vi "AU-EGSE Driver.vi"() -> ()   [LabVIEW 2025]
uses:
  <vilib>/Analysis/6fits.llb/Curve Fitting Criteria.ctl
  <vilib>/Analysis/1siggen.llb/Ramp Pattern by Samples.vi
  <vilib>/addons/_JKI Toolkits/State Machine/_JKI_lib_State_Machine.llb/Select State(s)_err__jki_lib_state_machine.vi
  <vilib>/Analysis/1siggen.llb/Ramp Pattern by Delta.vi
  <vilib>/Utility/file.llb/Write Delimited Spreadsheet (string).vi
  <vilib>/Utility/file.llb/Write Delimited Spreadsheet (DBL).vi
  <instrlib>/ULx/ULx_LV.dll
  <vilib>/Analysis/NI_AALBase.lvlib
  <userlib>/_OpenG.lib/time/time.llb/openg_time.lvlib
  <instrlib>/Detector SCPI/Detector SCPI.lvlib
  <instrlib>/Keithley 24XX/Keithley 24XX.lvlib
  <instrlib>/Keithley 648X Series/Keithley 648X Series.lvlib
  <vilib>/Analysis/NI_AALPro.lvlib
panel:
  in  "Exit":bool
  out "Searching":dbl[][](array[numeric])
  in  "Measurement Mode":T1(tab)=enum."SweepCurrent"
  in  "Connect PicoAmmeter":bool
  out "PicoAmmeter Connected":bool
  out "EGSE Connected":bool
  in  "Connect EGSE":bool
  in  "SPI Clock":i64=10000000 format="%^.0e"
  in  "Oversample":i32=1 min=1 max=4096
  in  "Board Power":bool
  in  "Detector VISA":refnum<visa-resource-name>="RS485_Comms"
  out "Voltage (V)":dbl[](array[numeric])=[0.0, 0.0, 0.0, 12.585]
  out "Current (mA)":dbl[](array[numeric])=[0.0, 0.0, 0.0, 0.915]
  in  "ThrowAway":i32=100 min=1 max=10000
  out "Detector EGSE ID String":string
  in  "B2901BL VISA":refnum<visa-resource-name>
  in  "Connect B2901BL":bool
  out "B2901BL Connected":bool
  in  "PicoAmmeter VISA":refnum<visa-resource-name>="Picoammeter"
  out "USB3104 Connected":bool
  in  "USB3104 VOut3 (SWIR)":refnum<k21>="Dev1/Ao3"
  in  "USB3104 VOut5 (MWIR)":refnum<k21>="Dev1/Ao3"
  in  "Connect USB3104":bool
  in  "Heater Power":bool
  in  "Vout3_Res":dbl=9993180.0 format="%#_4p"
  in  "Vout5_Res":dbl=9993180.0 format="%#_5p"
  in  "Set_SWIR":bool
  in  "MWIR Current":dbl
  in  "SWIR Current":dbl
  in  "ContGraph":enum32{"Science Packet", "Debug", "Temperature"}(tab)=enum."Temperature"
  in  "Export to Excel":bool
  out "All Counts":T2(graph)={"[0]"=0.0, "[1]"=0.0, "[2]"=0.0, "[3]"=0.0, "[4]"=0.0, "[5]"=0.0, "[6]"=0.0, "[7]"=0.0, "[8]"=0.0, "[9]"=889.63}
  out "Save FileName":string
  in  "test Results save directory":path
  in  "ResetScienceGraph":bool
  out "Averages":dbl[](array[numeric]) format="%#_3f"
  out "Counts":dbl(graph)
  out "Elapsed(uS)":i32=13
  out "Mean Value (counts)":dbl
  out "rms (counts) 2":dbl format="%^.4g"
  out "Peak-to-Peak (counts)":dbl format="%^.4g"
  in  "ResetVDACstats":bool
  out "Finding Offset...":bool
  in  "Find Offset":bool
  in  "Target Counts":i32=50 min=0 max=4095
  in  "Tolerance":dbl=10.0
  in  "Channel to Adjust":u16(ring) items=["SWIR", "MWIR"]
  in  "ADC Channel":u16(ring)=6 items=["SWIR:High", "SWIR:Med", "SWIR:Low", "MWIR:High", "MWIR:Med", "MWIR:Low", "TRP:HSink", "TRP:SWIR"]
  out "Board RTD Value Temperature":dbl(graph)=889.63
  in  "SWIR DAC":i32=2000 min=0 max=4095 step=1
  in  "MWIR DAC":i32=2000 min=0 max=4095 step=1
  in  "Timeout":i32=100
  in  "Set_MWIR":bool
  in  "Pause":bool
  out "XY Graph":cluster{dbl[], "subarray":dbl[]}(graph)
  in  "Pause Trigger":dbl=8.0 min=0.0 max=50.0
  in  "ADC Channel 2":u16(ring)=6 items=["SWIR:High", "SWIR:Med", "SWIR:Low", "MWIR:High", "MWIR:Med", "MWIR:Low", "TRP:HSink", "TRP:SWIR"]
  in  "MWIR sweep USB3104":bool
  in  "SWIR sweep USB3104":bool
  out "slope (counts/nA)":dbl
  out "intercept":dbl
  out "residue":dbl
  out "Max Deviation (counts)":dbl
  out "OutputCurrentGrph":cluster{"Ramp Pattern":dbl[], dbl[]}[](graph)
  in  "NumberDecades":i32=3
  in  "DecadeSweep":bool=TRUE
  in  "NPoints":i32=10 min=10 max=10000 step=1
  in  "MaxCurrent":dbl=1e-09 min=1e-11 max=1e-06
  in  "MinCurrent":dbl=1e-12 min=-10.0 max=10.0
  in  "B2901 Sweep":bool
  in  "NPointsPerDecade":u16(ring)=1 items=["1", "3", "9", "20"]
  out "Resistance (Ohms)":dbl
  out "IV Graph":cluster{"Ramp Pattern":dbl[], dbl[]}(graph)
  in  "NPoints 2":i32=10 min=10 max=10000 step=1
  in  "MaxVoltage":dbl=1e-09 min=0.0 max=10.0
  in  "MinVoltage":dbl=1e-12 min=0.0 max=10.0
  in  "Vout5 Sweep":bool
  in  "Vout3 Sweep":bool
  in  "Tab Control 2":enum32{"Science Mode", "Individual"}(tab)=enum."Individual"
  out "Count cs DAC":cluster{"X-Data":dbl[], "SciData":dbl[]}[](graph)
  out "VDAC Sweep":cluster{dbl[], dbl[]}[](graph)
  in  "SweepVDAC":bool
  in  "VDAC Step":i32=1 min=1 max=100
  in  "VDAC Max":i32 min=0 max=4095
  in  "VDAC Min":i32 min=0 max=4000
  in  "Channel to Sweep":u16(ring) items=["SWIR", "MWIR"]
  in  "Abort SweepVDAC":bool
  out "TRP Values":cluster{"output":i32, "output":i32}(graph)
  in  "DAC":i32 min=0 max=4095 step=1
  in  "Modulation Steps":i32=2 min=2 max=1000 step=1
  in  "Modulation Max":dbl min=0.0 max=10.0
  in  "Modulation Min":dbl min=-10.0 max=10.0
  in  "SweepLight":bool
  in  "Detector 7":u16(ring) items=["SWIR", "MWIR"]
  out "Output vs Light":cluster{dbl[], dbl[]}[](graph)
  in  "Gain 2":u16(ring) items=["High", "Med", "Low"]
  in  "Abort 2":bool
  out "Output vs Light 2":cluster{dbl[], dbl[]}[](graph)
  in  "StopGathering":bool=TRUE
  in  "Detector 2":u16(ring) items=["SWIR", "MWIR"]
  out "PhotoDiode":dbl
  in  "millisecond multiple":u32
  in  "Manual LightSweep":bool
  # "Instrument Connnections"
  # "ADC readout conditions"
  # "Detector Board and Heater Power"
  # "3.3V supply"
  # "Heater"
  # "+12V Supply"
  # "-12V Supply"
  # "NB. Voltage and current monitoring on heater circuit\nnot implemented in hardware."
  # "Resistor values for USB3104 based current source\nUpdated in \"Calibrate USB3104\""
  # "Read all 8 ADC channels in sequence according to current OS and Throwaway values. (ReadMode=\"Science\")  \nIPhoto is returned if picoammeter connected\nBoard Temp is returned from detector board TRP measured by EGSE"
  # "Read single ADC channel according to current OS and Throw values"
  # "Offset Autoadjust algorithm"
  # "Board Temperature returned by PRT on board read by EGSE"
  # "Pause button will halt collection and display.\nThis allows graph to be printed etc."
  # "Burst mode is intended to examine behaviour of the ADC\n\nA burst of readings is recorded on the EGSE and then gathered here.\n\"Throw\" readings are discarded and then \"Oversample\" readings\ndirect from selected ADC into EGSE buffer and displayed."
  # "Record output as photodiode input is swept over range set up.\nData is recorded as per science packet formation, whereby each channel is read according to throw/oversample settings before moving on to the next xhannel.\nCurrent source for sweep is either Keithley B2901BL connected to appropriate input or using Vout3 and VOut5 from USB3104 pod with appropriate seies resistors."
  # "Place cursors on chart to extract slope & offset"
  # "Sweeps USB3104 voltage output and records current on 6485 picoammeter allowing value for series resistor to be determined."
  # "Resistance determined from slope of graph"
  # "Data taken from all 8 ADC channels as per current throw and OS parameters"
  # "Data taken from just 3 ADC inputs on current channel as per current throw and OS parameters"
  # "Light source modulated by USB205L working as voltage source connected to MOD input of LD250C\nreference photodiode monitored by 6846 picoammeter"
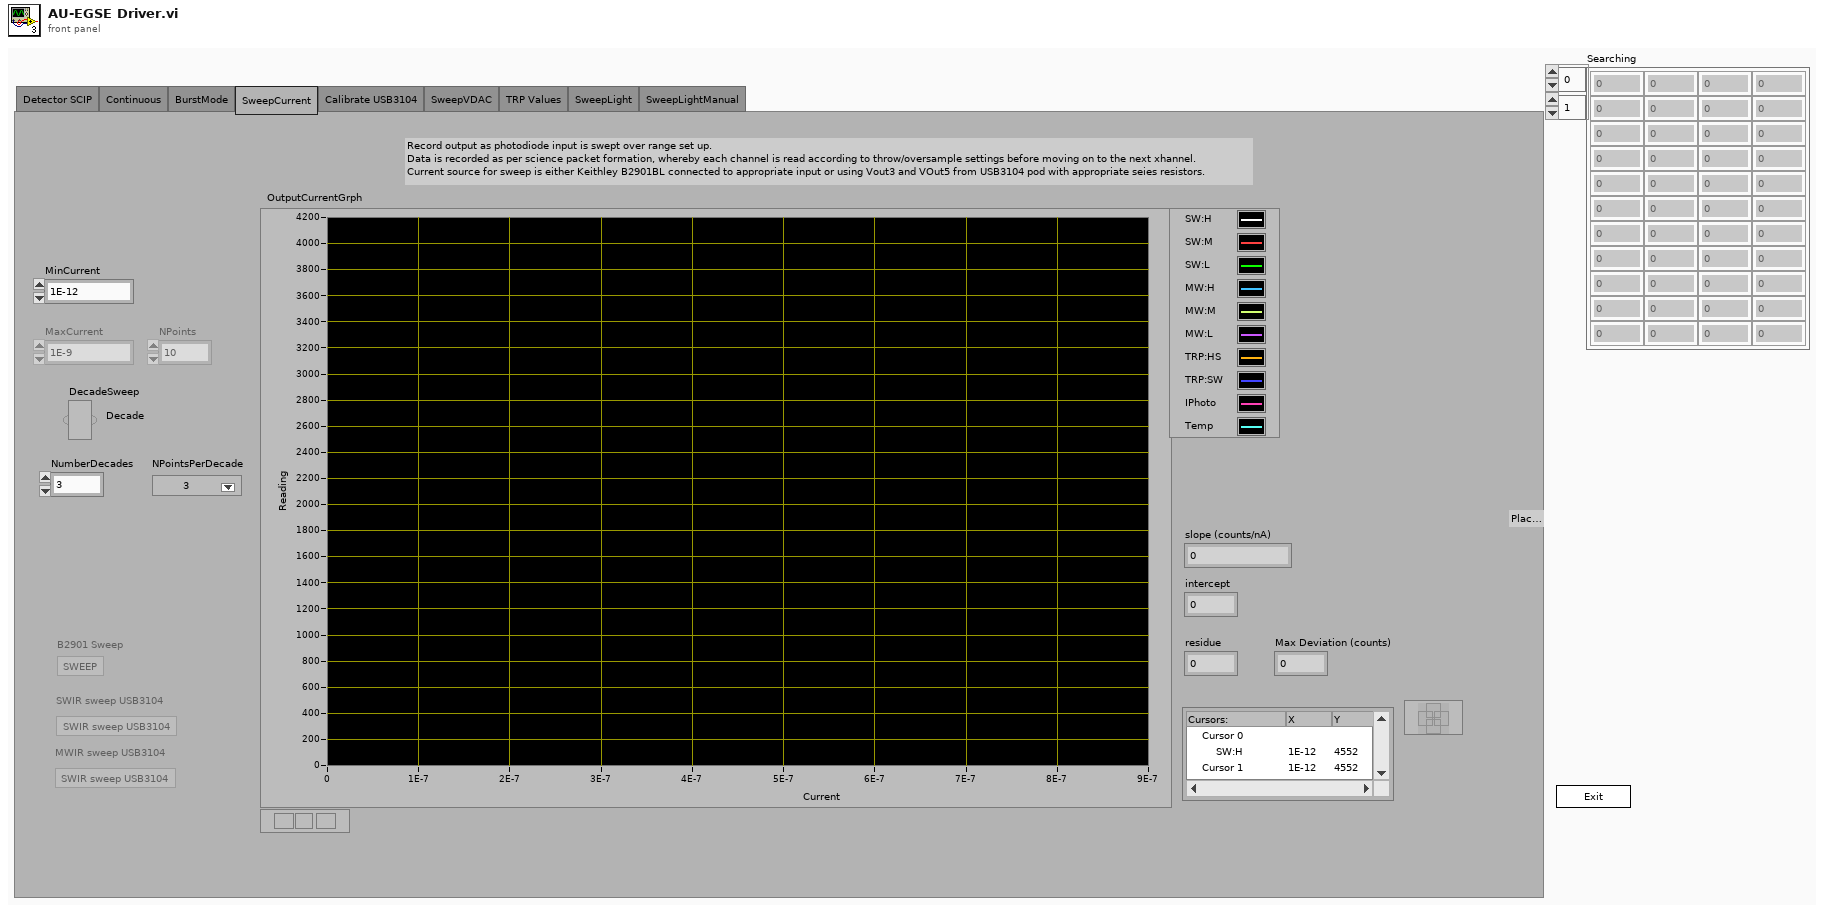
[diagram p1: front panel]
types:
  T1 = enum32{"Detector SCIP", "Continuous", "BurstMode", "SweepCurrent", "Calibrate USB3104", "SweepVDAC", "TRP Values", "SweepLight", "SweepLightManual"}
  T2 = cluster{"[0]":dbl, "[1]":dbl, "[2]":dbl, "[3]":dbl, "[4]":dbl, "[5]":dbl, "[6]":dbl, "[7]":dbl, "[8]":dbl, "[9]":dbl}
  T3 = cluster{"[0]":dbl, "[1]":dbl, "[2]":dbl, "[3]":dbl, "[4]":dbl, "[5]":dbl, "[6]":dbl, "[7]":dbl, "[8]":dbl, "[9]":dbl}[]
  T4 = enum32{"Invalid", "Standard", "Closed", "Hidden", "Minimized", "Maximized"}
  T5 = enum32{"invalid app kind", "Development System", "Run Time System", "Student Edition", "Embedded LabVIEW", "Evaluation", "Custom"}
  T6 = enum8{"Enabled", "Disabled", "Disabled and Grayed Out"}
  T7 = cluster{"Baud Rate":u32, "Parity":u16, "Data Bits":u16, "Stop Bits":u16, "Flow Control":u16}
  T8 = cluster{"Core":cluster{"Current VI Reference":refnum<vi>, "Close Panel on Exit?":bool}, "Detector Resource":refnum<visa-resource-name>, "EGSE connected":bool, "PicoAmmeter Resource":refnum<visa-resource-name>, "Picoammeter connected":bool, "B2901 Resource":refnum<visa-resource-name>, "B2901 connected":bool, "SWIR CurrentSource":refnum<k24>, "MWIR CurrentSource":refnum<k24>, "USB3104 connected":bool, "OpVsCurrent":cluster{"Ramp Pattern":dbl[], dbl[]}[], "Vout3_Res":dbl, "Vout5_Res":dbl}
  T9 = typedef "NI_AALPro.lvlib/Curve Fitting Criteria.ctl" = u16
  T10 = typedef "LVPointDoubleTypeDef.ctl" = cluster{"Cursor X":dbl, "Cursor Y":dbl}
  T11 = cluster{"Current VI Reference":refnum<vi>, "Close Panel on Exit?":bool}
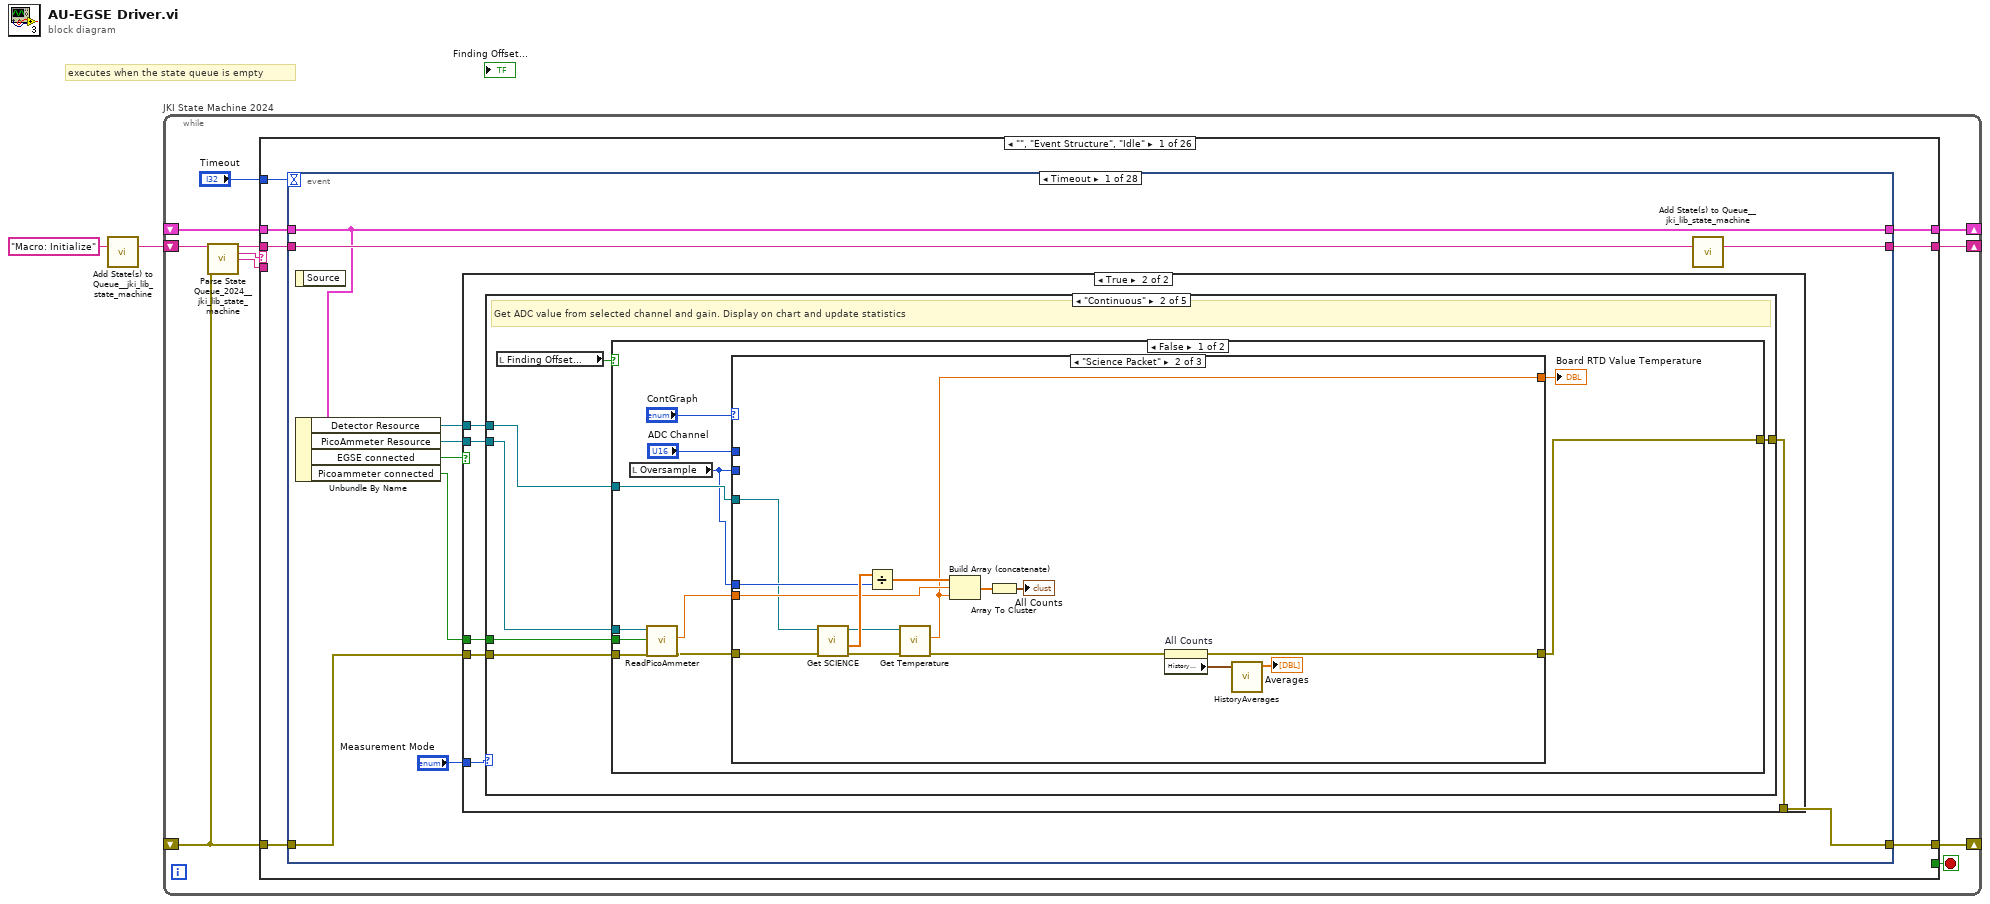
[diagram p0: block diagram]
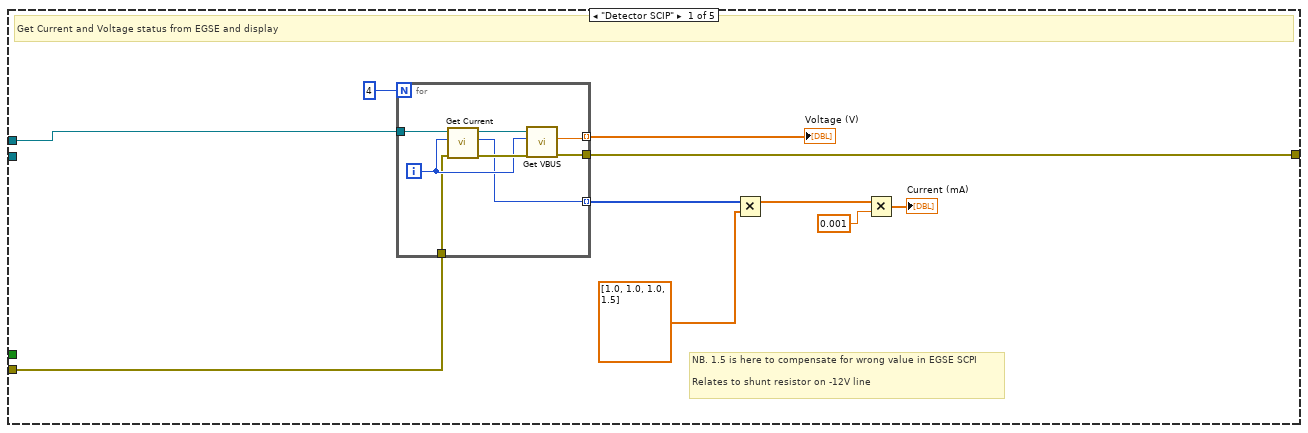
[diagram p3: hidden frame]
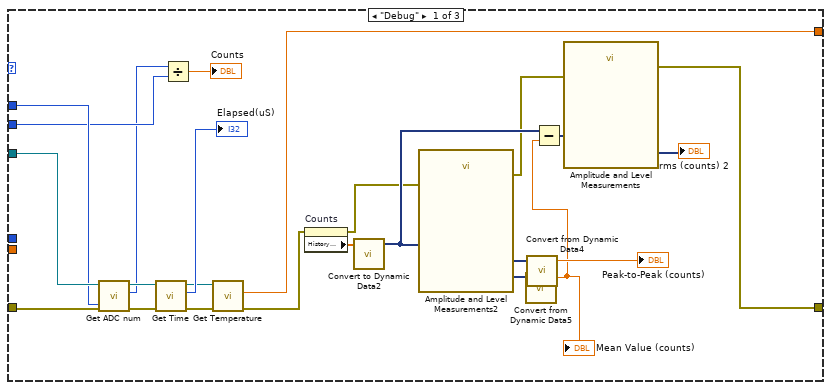
[diagram p4: hidden frame]
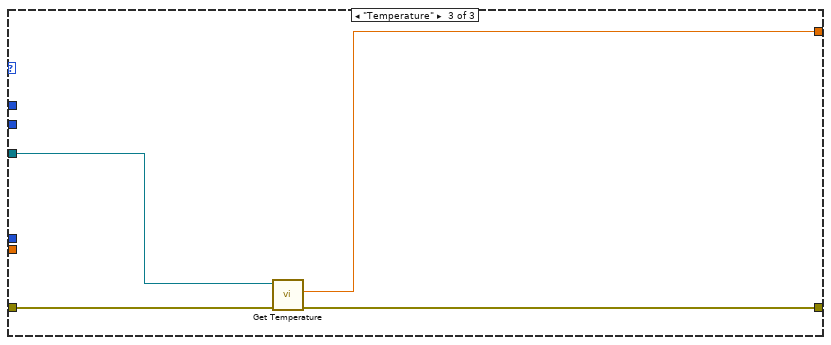
[diagram p5: hidden frame]
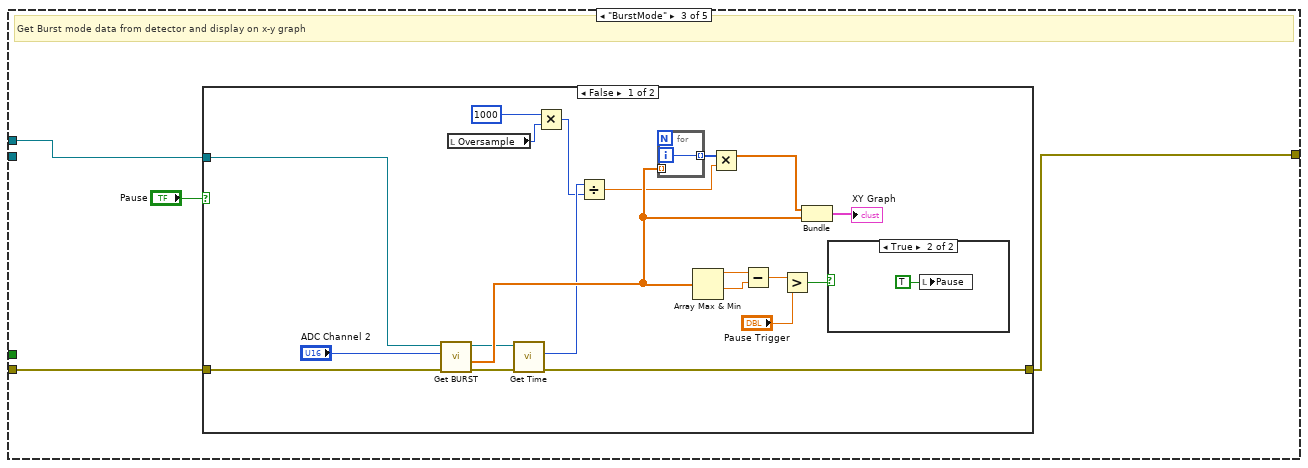
[diagram p7: hidden frame]
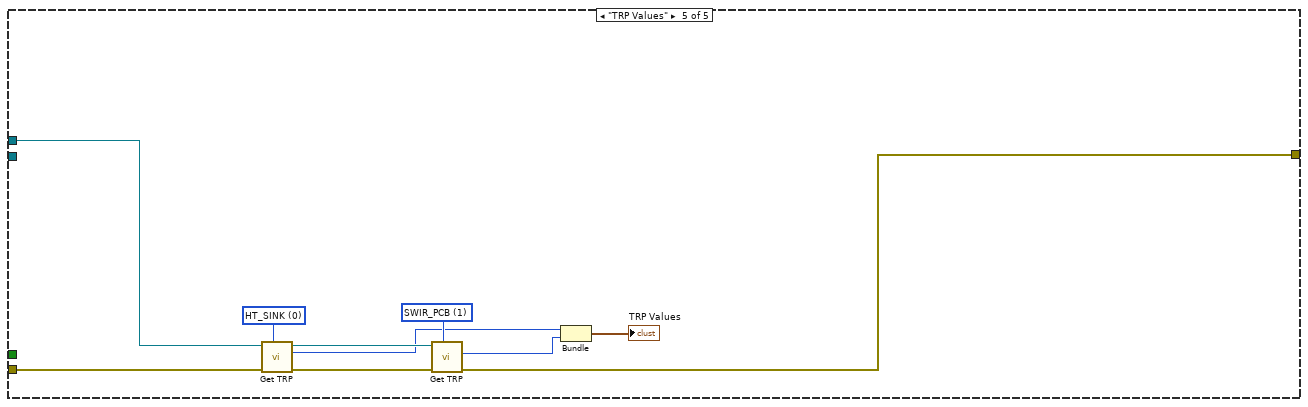
[diagram p11: hidden frame]
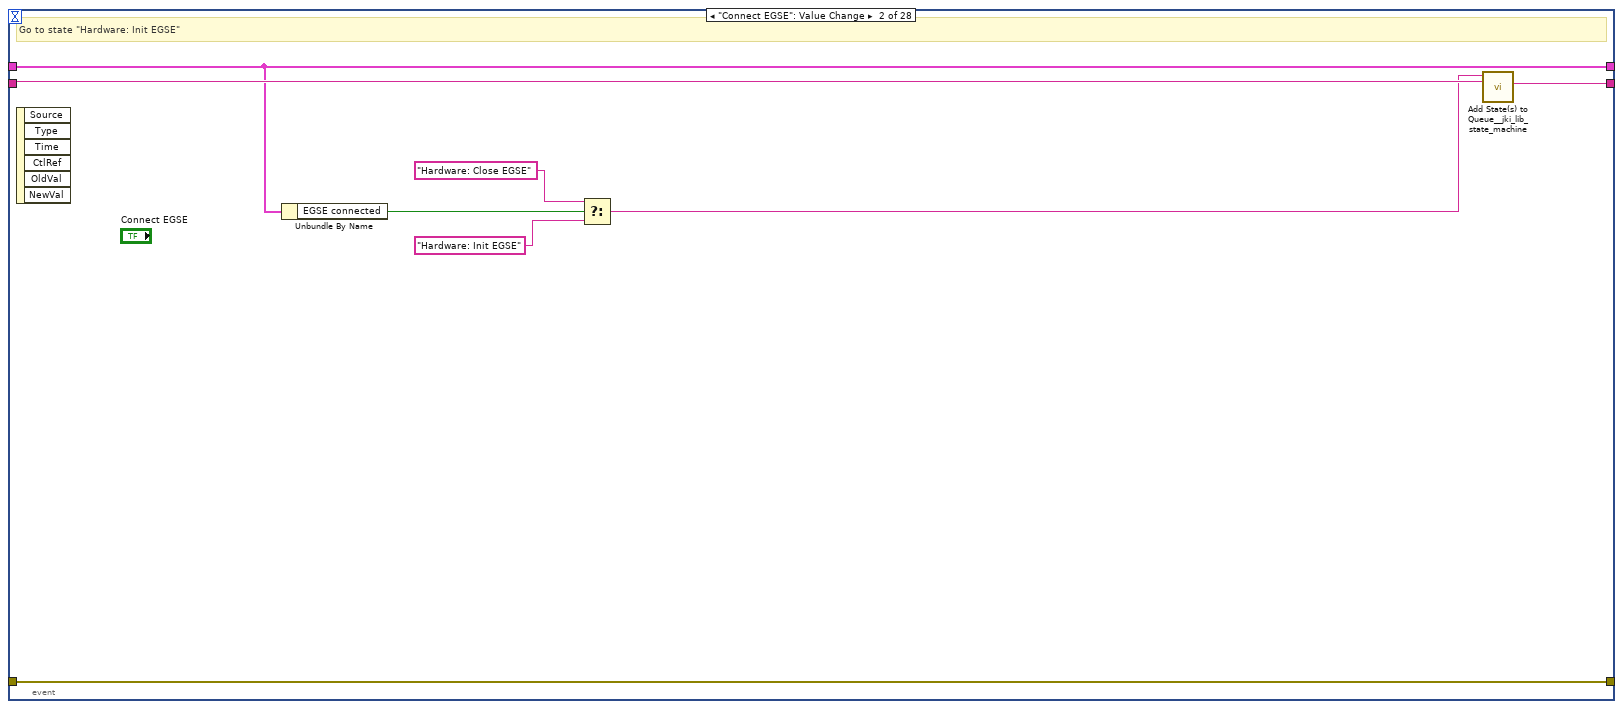
[diagram p12: hidden frame]
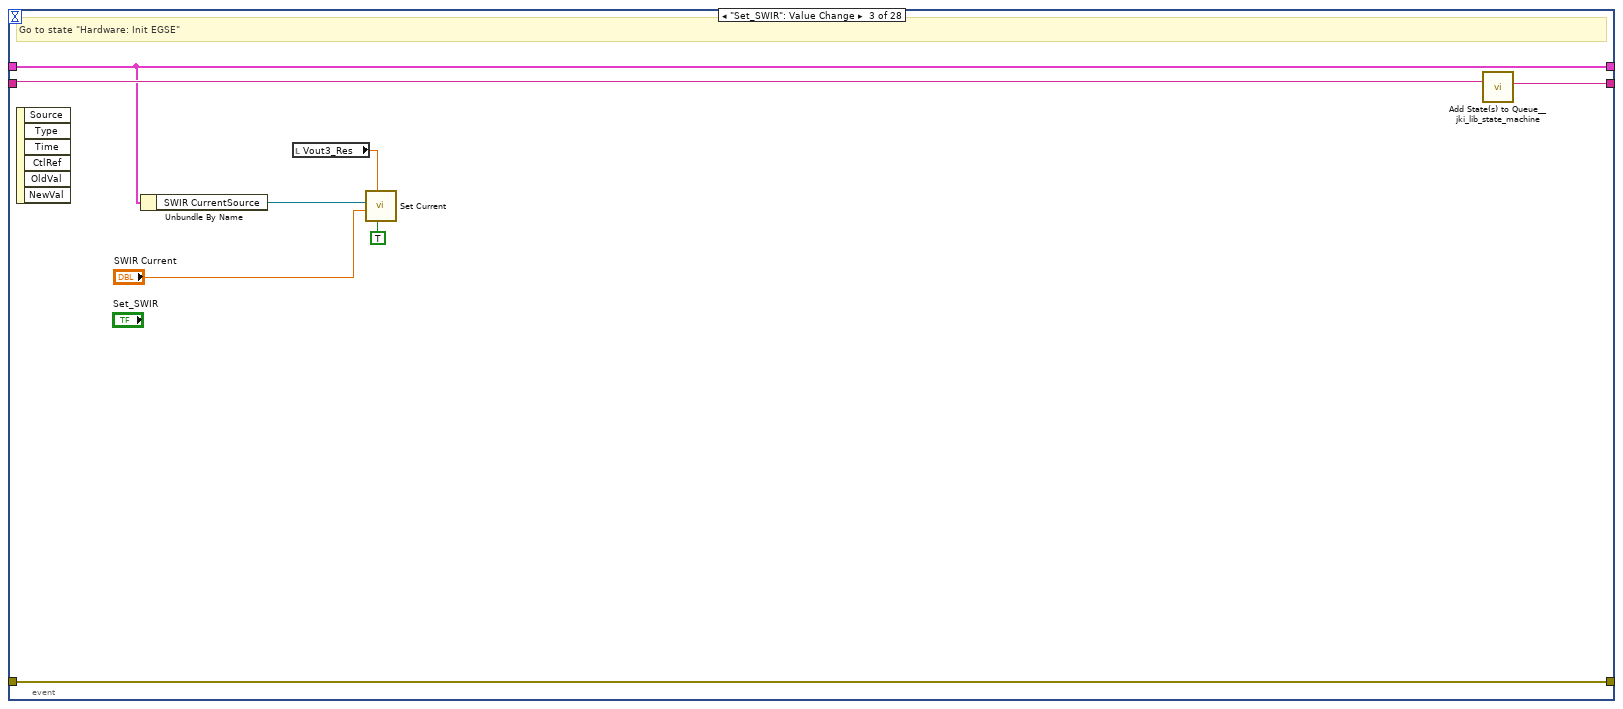
[diagram p13: hidden frame]
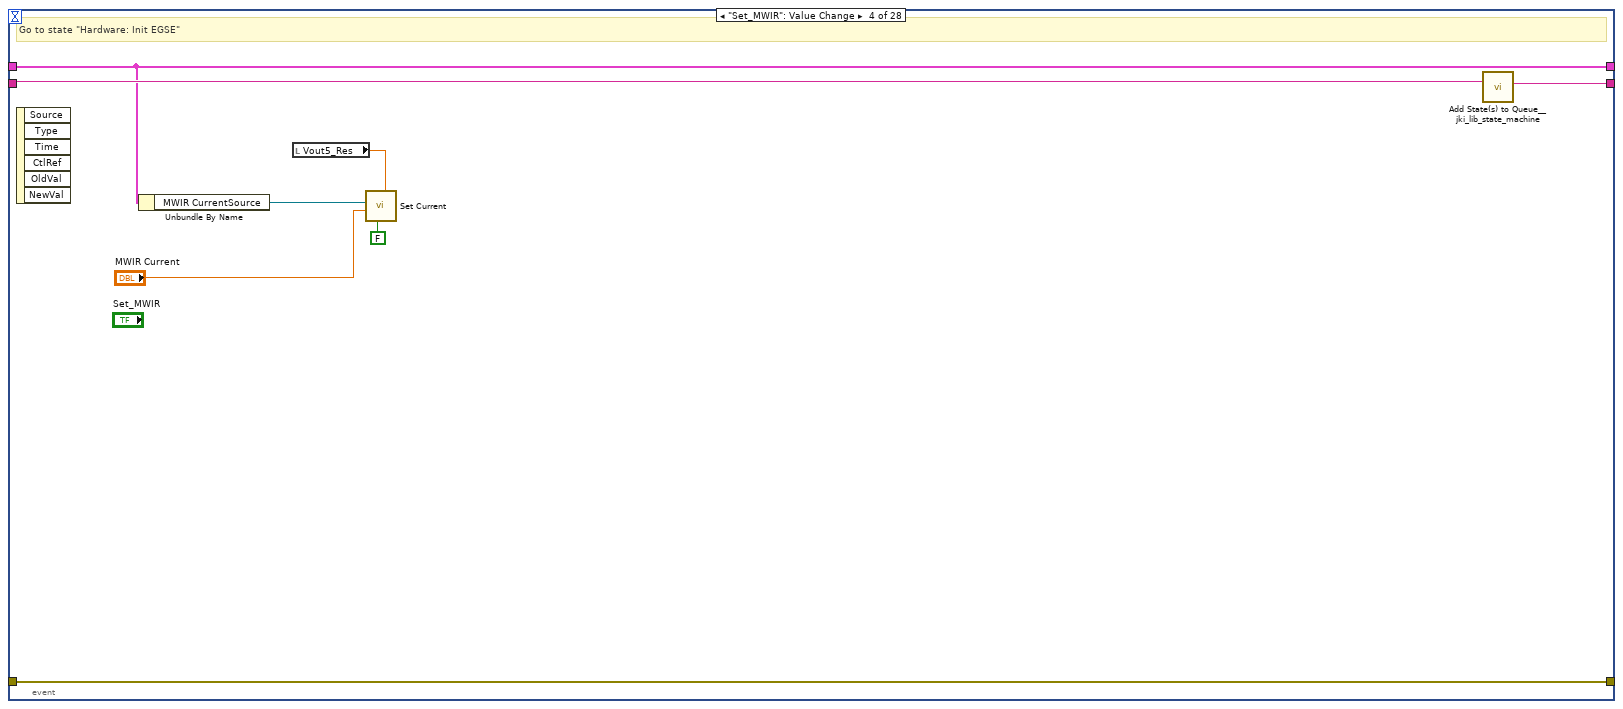
[diagram p14: hidden frame]
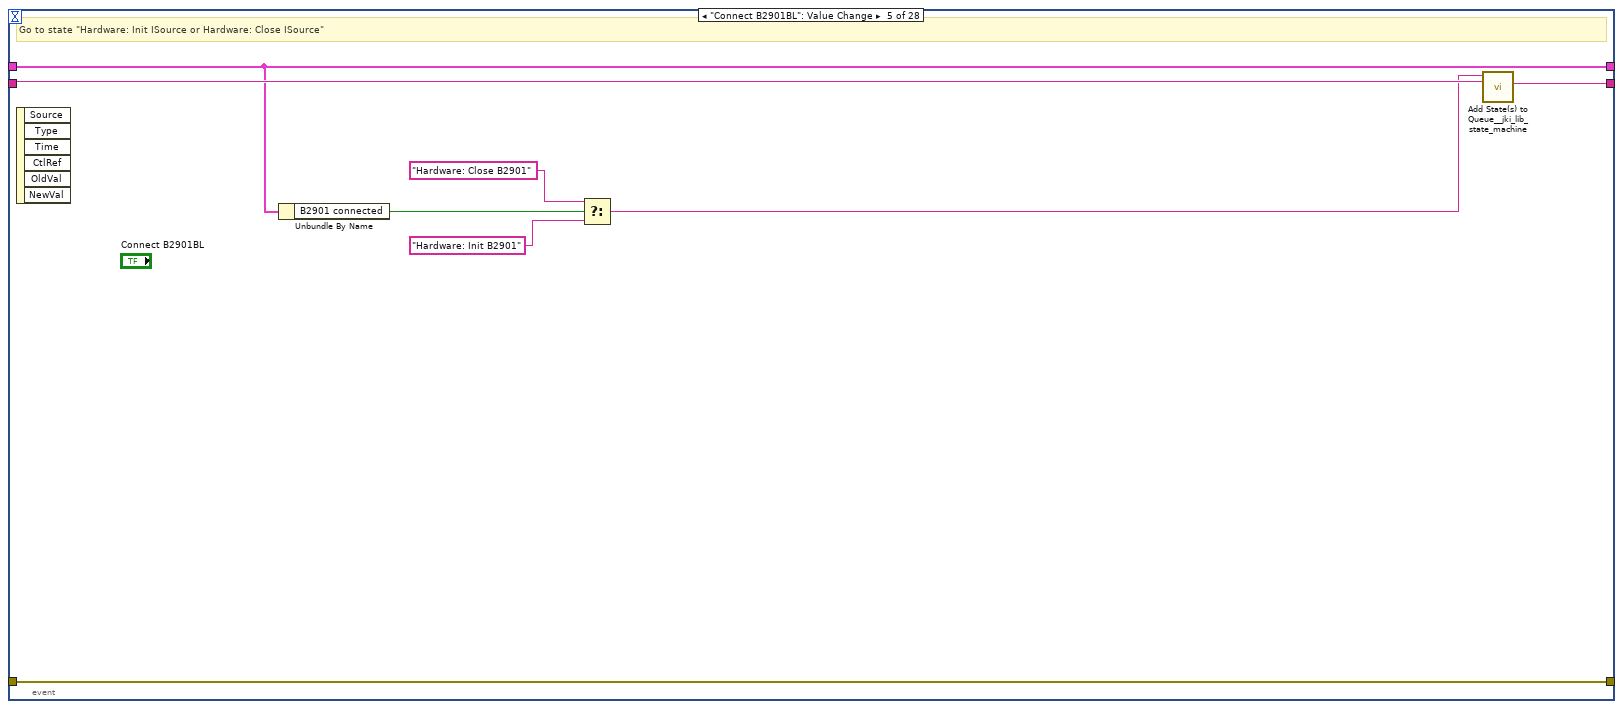
[diagram p15: hidden frame]
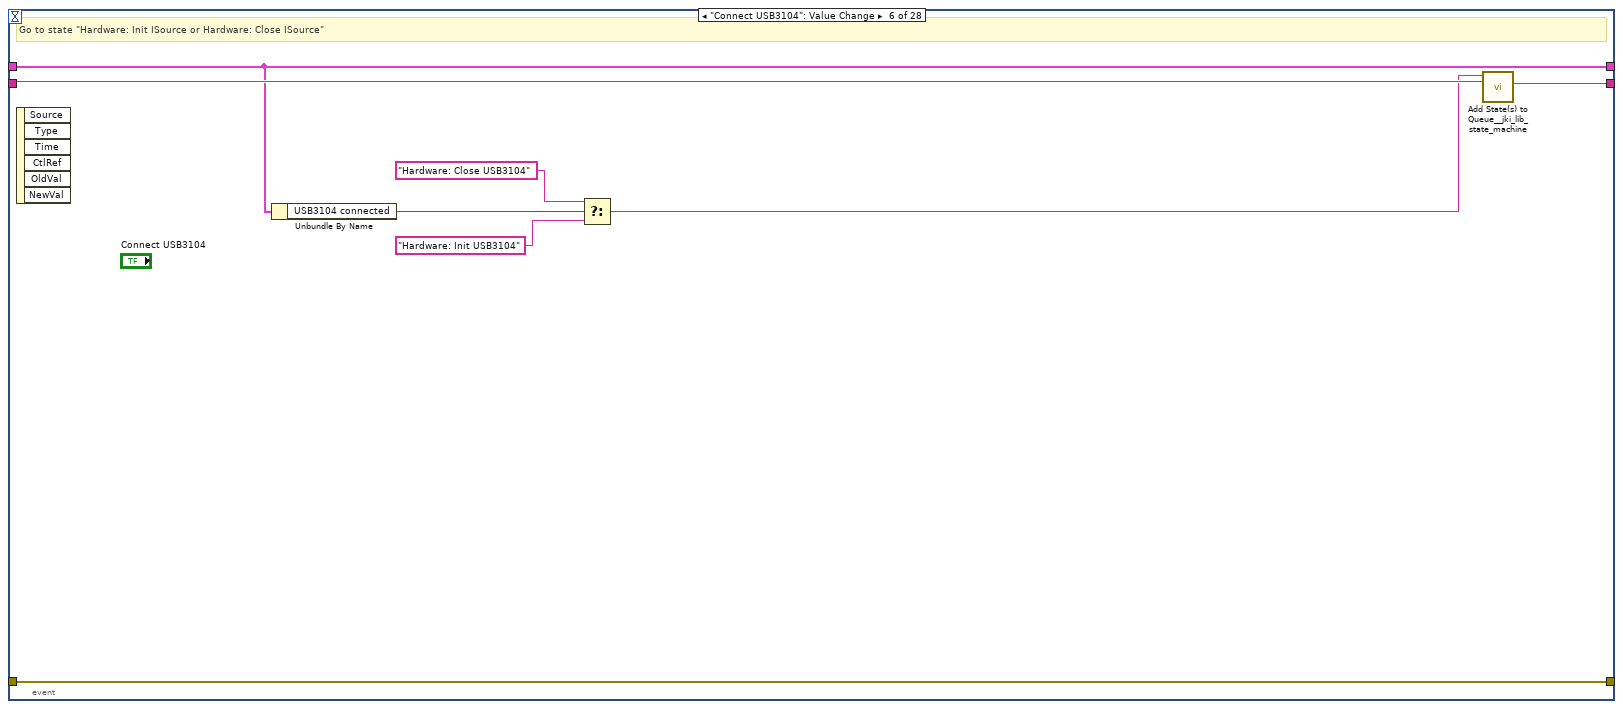
[diagram p16: hidden frame]
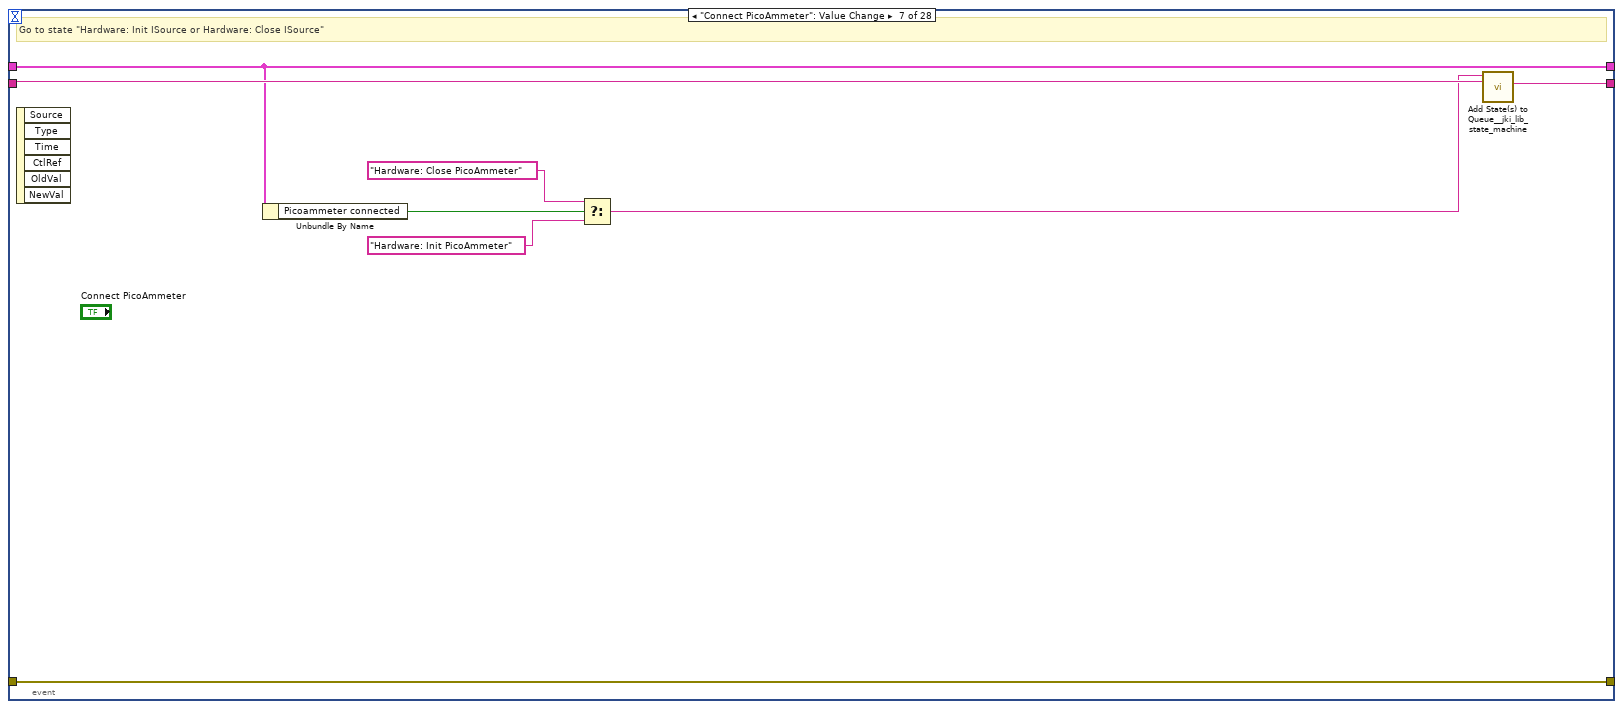
[diagram p17: hidden frame]
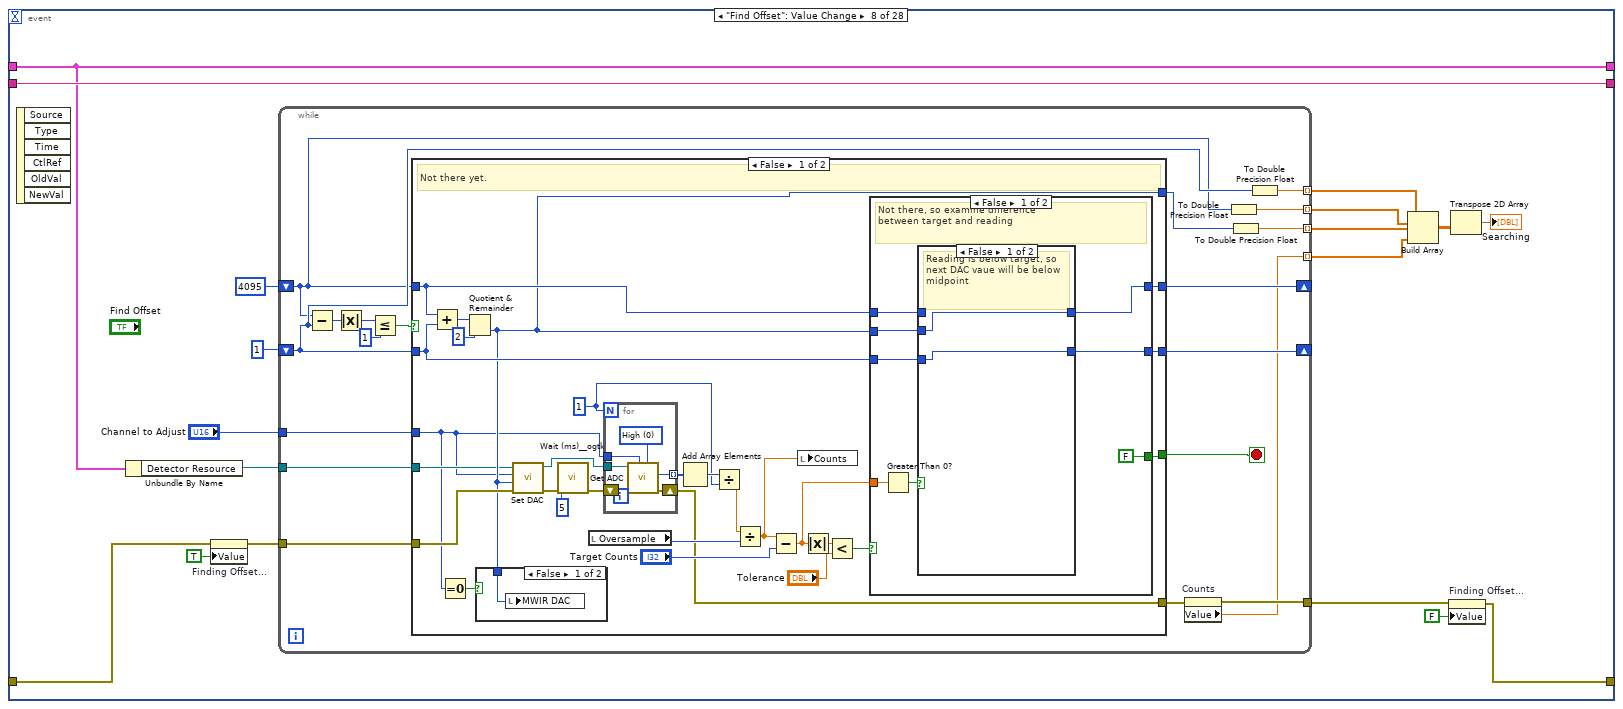
[diagram p18: hidden frame]
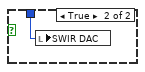
[diagram p19: hidden frame]
diagram:
  # "executes when the state queue is empty"
  n1 = call <vilib>:"Add State(s) to Queue__jki_lib_state_machine.vi"("State(s) in (\"\")"="Macro: Initialize") -> ("States Out"=w2:string)  [unwired: 14 in]
  n2 = while "JKI State Machine 2024" {
    shift-right: [w6] -> _
    shift-left: _ -> [w5]
    shift-right: [w9] -> _
    shift-left: _ -> [w3]
    shift-right: [w8] -> _
    shift-left: w2 -> [w10]
    stop <- w7 stop-if-true
    n3 = call <vilib>:"Parse State Queue_2024__jki_lib_state_machine.vi"("State Queue"=w10, "Error In (no error)"=w3) -> ("Remaining States"=w12:string, "Current State"=w13:string, "Arguments"=w11:string)  [unwired: 11 in]
    n4 = case shown="\"\", \"Event Structure\", \"Idle\"" w13 {
      selector: w13 -> [_ _ w867 _ _ _ _ _ _ _ _ _ _ _ _ _ _ _ _ _ _ _ _ _ _ _]
      tunnel: w12 -> [w20 w866 w871 w890 w900 w909 w913 w930 w936 w940 w950 w958 w964 w975 w1044 w1049 w1058 w1062 w1071 w1091 w1139 w1162 w1197 w1228 w1246 w1274]
      tunnel: w11 -> [_ _ _ _ w895 _ _ _ _ _ _ _ w959 w969 _ _ _ _ _ _ _ _ _ _ _ _]
      tunnel: w5 -> [w18 w863 w869 w883 w897 w907 w910 _ w931 w937 w948 w956 w962 w971 w1041 w1046 w1056 w1059 w1066 w1089 w1137 w1153 w1193 w1224 w1244 w1272]
      tunnel: [w17 w864 w873 w887 errorcluster {"status"=FALSE, "code"=0, "source"=""} ("error out") w906 w911 w927 w932 w938 w947 w955 w960 w972 w1042 w1047 w1053 w1060 w1063 w1082 w1135 w1156 w1191 w1222 w1243 w1270] -> w9
      tunnel: w3 -> [w14 w864 w872 w887 w896 w906 w911 w927 w933 w938 w947 w955 w961 w973 w1042 w1047 w1053 w1060 w1068 w1084 w1134 w1155 w1195 w1226 w1242 w1269]
      tunnel: [w19 w865 w870 w889 w899 w908 w912 w929 w935 w939 w949 w957 w963 w974 w1043 w1048 w1057 w1061 w1070 w1090 w1138 w1161 w1196 w1227 w1245 w1273] -> w8
      tunnel: [_ _ _ _ _ TRUE _ _ _ _ _ _ _ _ _ _ _ _ _ _ _ _ _ _ _ _] -> w7
      tunnel: [w16 w863 w869 w888 w897 w907 w910 w928 w931 w937 w948 w956 w962 w971 w1041 w1046 w1056 w1059 w1065 w1086 w1136 w1152 w1192 w1223 w1239 w1271] -> w6
      tunnel: "Timeout" -> [w15 _ _ _ _ _ _ _ _ _ _ _ _ _ _ _ _ _ _ _ _ _ _ _ _ _]
      frame "", "Event Structure", "Idle" {
        n5 = event shown="[0] Timeout" {
          selector: _ -> [_ _ _ _ _ _ _ _ _ _ _ _ _ _ _ _ _ _ _ _ _ _ _ _ _ _ _ _]
          dyn-events: _ -> [_ _ _ _ _ _ _ _ _ _ _ _ _ _ _ _ _ _ _ _ _ _ _ _ _ _ _ _]
          timeout: w15 -> [_ _ _ _ _ _ _ _ _ _ _ _ _ _ _ _ _ _ _ _ _ _ _ _ _ _ _ _]
          tunnel: w20 -> [w30 w160 w168 w176 w184 w192 w200 w206 w295 w306 w313 w319 w324 w377 w458 w464 w468 w472 w479 w507 w518 w602 w682 w747 w751 w789 w856 w862]
          tunnel: [w29 w161 w169 w177 w185 w193 w201 w206 w295 w306 w313 w319 w324 w377 w458 w464 w468 w472 w479 w507 w518 w602 w682 w747 w751 w789 w855 w861] -> w19
          tunnel: w18 -> [w25 w159 w167 w175 w183 w191 w199 w204 w296 w304 w312 w318 w320 w374 w456 w462 w469 w473 w480 w505 w510 w592 w673 w746 w750 w787 w853 w859]
          tunnel: [w26 w162 w170 w178 w186 w194 w202 w207 w294 w302 w310 w316 w321 w375 w457 w463 w470 w474 w477 w508 w515 w599 w680 w748 w752 w784 w854 w860] -> w17
          tunnel: w14 -> [w27 w162 w170 w178 w186 w194 w202 w208 w294 w303 w309 w315 w322 w376 w457 w463 w470 w474 w478 w508 w516 w600 w681 w748 w752 w785 w854 w860]
          tunnel: [w25 w159 w167 w175 w183 w191 w199 w204 w296 w304 w312 w318 w320 w374 w456 w462 w469 w473 w480 w505 w509 w591 w672 w746 w750 w787 w853 w859] -> w16
          event Timeout {
            n6 = event-data() -> ()  [unwired: 1 in, 1 out]
            n7 = Unbundle By Name(w25) -> ("Detector Resource"=w24:refnum<visa-resource-name>, "PicoAmmeter Resource"=w23:refnum<visa-resource-name>, "EGSE connected"=w22:bool, "Picoammeter connected"=w21:bool)
            n8 = case shown="True" w22 {
              tunnel: "Measurement Mode" -> [_ w37]
              tunnel: w27 -> [w31 w36]
              tunnel: [w31 w35] -> w26
              tunnel: w24 -> [_ w34]
              tunnel: w23 -> [_ w33]
              tunnel: w21 -> [_ w32]
              frame False {
              }
              frame True {
                n9 = case shown="\"Continuous\"" w37 {
                  tunnel: w36 -> [w40 w59 w119 w144 w147]
                  tunnel: [w39 w57 w118 w144 w146] -> w35
                  tunnel: w34 -> [w38 w60 w117 _ w148]
                  tunnel: w33 -> [_ w58 _ _ _]
                  tunnel: w32 -> [_ w56 _ _ _]
                  frame "Detector SCIP" {
                    # "NB. 1.5 is here to compensate for wrong value in EGSE SCPI\n\nRelates to shunt resistor on -12V line"
                    # "Get Current and Voltage status from EGSE and display"
                    n10 = for {
                      N: 4 -> [_]
                      tunnel: w38 -> [w48]
                      tunnel: [w52] -> w45 mode=indexing
                      tunnel: [w51] -> w46 mode=indexing
                      tunnel: [w50] -> w39
                      tunnel: w40 -> [w49]
                      i -> [w53]
                      n11 = call <instrlib>:"Get Current.vi"("error in (no error)"=w49, "chan (1)"=w53, "VISA resource name"=w48) -> ("error out"=w55:errorcluster, "output"=w52:i32, "VISA resource name out"=w54:refnum<visa-resource-name>)  [unwired: 6 in]
                      n12 = call <instrlib>:"Get VBUS.vi"("error in (no error)"=w55, "chan (1)"=w53, "VISA resource name"=w54) -> ("error out"=w50:errorcluster, "output"=w51:dbl)  [unwired: 6 in, 1 out]
                    }
                    "Voltage (V)" <- w46
                    n13 = Multiply(x=w45, y=dbl[] [1.0, 1.0, 1.0, 1.5]) -> (x*y=w42:dbl[])
                    n14 = Multiply(x=w42, y=0.001) -> (x*y=→"Current (mA)":dbl[])
                  }
                  frame "Continuous" {
                    # "Get ADC value from selected channel and gain. Display on chart and update statistics"
                    n15 = local read "Finding Offset..."() -> (w61:bool)
                    n16 = case shown="False" w61 {
                      tunnel: w60 -> [w71 _]
                      tunnel: w59 -> [w69 w116]
                      tunnel: w58 -> [w70 _]
                      tunnel: [w62 w116] -> w57
                      tunnel: w56 -> [w66 _]
                      frame False {
                        n17 = local read "Oversample"() -> (w63:i32)
                        n18 = call "ReadPicoAmmeter.vi"("error in (no error)"=w69, "Connected"=w66, "PicoAmmeter"=w70) -> ("error out"=w68:errorcluster, "Current"=w67:dbl)  [unwired: 7 in]
                        n19 = case shown="\"Science Packet\"" "ContGraph" {
                          tunnel: w71 -> [w95 w102 w112]
                          tunnel: "ADC Channel" -> [w91 _ _]
                          tunnel: w63 -> [_ w108 _]
                          tunnel: w68 -> [w96 w107 w113]
                          tunnel: w67 -> [_ w105 _]
                          tunnel: [w73 w99 w115] -> w62
                          tunnel: [w89 w101 w114] -> w64
                          tunnel: w63 -> [w86 _ _]
                          frame "Debug" {
                            n20 = call <instrlib>:"Get ADC num.vi"("Channel"=w91, "error in (no error)"=w96, "VISA resource name"=w95) -> ("error out"=w92:errorcluster, "output"=w85:i32, "VISA resource name out"=w93:refnum<visa-resource-name>)  [unwired: 6 in]
                            n21 = call <instrlib>:"Get Time.vi"("error in (no error)"=w92, "VISA resource name"=w93) -> ("error out"=w90:errorcluster, "output"=→"Elapsed(uS)":i32, "VISA resource name out"=w88:refnum<visa-resource-name>)  [unwired: 7 in]
                            n22 = Divide(x=w85, y=w86) -> (x/y=→"Counts":dbl)
                            n23 = call "Get Temperature.vi"("error in (no error)"=w90, "VISA resource name"=w88) -> ("error out"=w75:errorcluster, "output"=w89:dbl)  [unwired: 7 in, 1 out]
                            n24 = property on="Counts" class="WFChart (strict)"(error in=w75) -> (error out=w74:errorcluster, "History Data"=w77:dbl[])  [unwired: 1 in, 1 out]
                            n25 = call "Convert to Dynamic Data2"("Array"=w77) -> ("Dynamic Data Type"=w78:dynamicdata)  [unwired: 3 in]
                            n26 = call "Amplitude and Level Measurements2"("Signals"=w78, "error in (no error)"=w74) -> ("Mean (DC)"=w80:dynamicdata, "Peak to Peak"=w83:dynamicdata, "error out"=w76:errorcluster)  [unwired: 10 in, 1 out]
                            n27 = call "Convert from Dynamic Data5"("Dynamic Data Type"=w80) -> ("Scalar"=w79:dbl)  [unwired: 3 in]
                            "Mean Value (counts)" <- w79
                            n28 = call "Convert from Dynamic Data4"("Dynamic Data Type"=w83) -> ("Scalar"=→"Peak-to-Peak (counts)":dbl)  [unwired: 3 in]
                            n29 = Subtract(x=w78, y=w79) -> (x-y=w81:dynamicdata)
                            n30 = call "Amplitude and Level Measurements"("Signals"=w81, "error in (no error)"=w76) -> ("RMS"=→"rms (counts) 2":dynamicdata, "error out"=w73:errorcluster)  [unwired: 10 in, 2 out]
                          }
                          frame "Science Packet" {
                            n31 = call <instrlib>:"Get SCIENCE.vi"("error in (no error)"=w107, "VISA resource name"=w102) -> ("error out"=w104:errorcluster, "subarray"=w109:dbl[], "VISA resource name out"=w103:refnum<visa-resource-name>)  [unwired: 6 in, 1 out]
                            n32 = Divide(x=w109, y=w108) -> (x/y=w110:dbl[])
                            n33 = call "Get Temperature.vi"("error in (no error)"=w104, "VISA resource name"=w103) -> ("error out"=w100:errorcluster, "output"=w101:dbl)  [unwired: 7 in, 1 out]
                            n34 = Build Array (concatenate)(w110, w105, w101) -> (w106:dbl[])
                            n35 = Array To Cluster(array=w106) -> (cluster=→"All Counts":T2)
                            n36 = property on="All Counts" class="WFChart (strict)"(error in=w100) -> (error out=w99:errorcluster, "History Data"=w98:T3)  [unwired: 1 in, 1 out]
                            n37 = call "HistoryAverages.vi"("History Data"=w98) -> ("Averages"=→"Averages":dbl[])  [unwired: 10 in]
                          }
                          frame "Temperature" {
                            n38 = call "Get Temperature.vi"("error in (no error)"=w113, "VISA resource name"=w112) -> ("error out"=w115:errorcluster, "output"=w114:dbl)  [unwired: 7 in, 1 out]
                          }
                        }
                        "Board RTD Value Temperature" <- w64
                      }
                      frame True {
                      }
                    }
                  }
                  frame "BurstMode" {
                    # "Get Burst mode data from detector and display on x-y graph"
                    n39 = case shown="False" "Pause" {
                      tunnel: w119 -> [w124 w143]
                      tunnel: [w123 w143] -> w118
                      tunnel: w117 -> [w122 _]
                      frame False {
                        n40 = call <instrlib>:"Get BURST.vi"("error in (no error)"=w124, "chan (0)"="ADC Channel 2", "VISA resource name"=w122) -> ("error out"=w132:errorcluster, "subarray"=w138:dbl[], "VISA resource name out"=w131:refnum<visa-resource-name>)  [unwired: 5 in, 1 out]
                        n41 = local read "Oversample"() -> (w130:i32)
                        n42 = call <instrlib>:"Get Time.vi"("error in (no error)"=w132, "VISA resource name"=w131) -> ("error out"=w123:errorcluster, "output"=w129:i32)  [unwired: 7 in, 1 out]
                        n43 = Multiply(x=1000, y=w130) -> (x*y=w126:i32)
                        n44 = Divide(x=w129, y=w126) -> (x/y=w127:dbl)
                        n45 = for {
                          tunnel: w138 -> [_] mode=indexing
                          tunnel: [w142] -> w139 mode=indexing
                          i -> [w142]
                        }
                        n46 = Array Max & Min(array=w138) -> (max value=w137:dbl, min value=w136:dbl)  [unwired: 2 out]
                        n47 = Multiply(x=w139, y=w127) -> (x*y=w128:dbl[])
                        n48 = Subtract(x=w137, y=w136) -> (x-y=w135:dbl)
                        n49 = Greater?(x=w135, y="Pause Trigger") -> (0:w133:bool)
                        n50 = Bundle(w128, "subarray"=w138) -> (→"XY Graph":cluster{dbl[], "subarray":dbl[]})  [unwired: 1 in]
                        n51 = case shown="True" w133 {
                          frame False {
                          }
                          frame True {
                            n52 = local write "Pause"(TRUE ("Pause")) -> ()
                          }
                        }
                      }
                      frame True {
                      }
                    }
                  }
                  frame "SweepCurrent", Default {
                  }
                  frame "TRP Values" {
                    w145 = u16 0 items=["HT_SINK", "SWIR_PCB"] ("TRP")
                    w153 = u16 1 items=["HT_SINK", "SWIR_PCB"] ("TRP")
                    n53 = call <instrlib>:"Get TRP.vi"("TRP"=w145, "error in (no error)"=w147, "VISA resource name"=w148) -> ("error out"=w152:errorcluster, "output"=w151:i32, "VISA resource name out"=w154:refnum<visa-resource-name>)  [unwired: 6 in]
                    n54 = call <instrlib>:"Get TRP.vi"("TRP"=w153, "error in (no error)"=w152, "VISA resource name"=w154) -> ("error out"=w146:errorcluster, "output"=w150:i32)  [unwired: 6 in, 1 out]
                    n55 = Bundle("output"=w151, "output"=w150) -> (→"TRP Values":cluster{"output":i32, "output":i32})  [unwired: 1 in]
                  }
                }
              }
            }
            n56 = call <vilib>:"Add State(s) to Queue__jki_lib_state_machine.vi"("State(s) in (\"\")"=w30) -> ("States Out"=w29:string)  [unwired: 14 in]
          }
          event "Connect EGSE": Value Change {
            # "Go to state \"Hardware: Init EGSE\""
            n57 = event-data() -> ()  [unwired: 1 in, 6 out]
            n58 = Unbundle By Name(w159) -> ("EGSE connected"=w158:bool)
            n59 = Select(t="Hardware: Close EGSE", s=w158, f="Hardware: Init EGSE" ("State(s) in Front (\"\")")) -> (s? t:f=w156:string)
            n60 = call <vilib>:"Add State(s) to Queue__jki_lib_state_machine.vi"("State(s) in Front (\"\")"=w156, "State(s) in (\"\")"=w160) -> ("States Out"=w161:string)  [unwired: 13 in]
          }
          event "Set_SWIR": Value Change {
            # "Go to state \"Hardware: Init EGSE\""
            n61 = event-data() -> ()  [unwired: 1 in, 6 out]
            n62 = Unbundle By Name(w167) -> ("SWIR CurrentSource"=w166:refnum<k24>)
            n63 = local read "Vout3_Res"() -> (w163:dbl)
            n64 = call "Set Current.vi"("SWIR?"=TRUE, "Vout3_Res"=w163, "Current"="SWIR Current", "task in"=w166) -> ()  [unwired: 6 in, 2 out]
            n65 = call <vilib>:"Add State(s) to Queue__jki_lib_state_machine.vi"("State(s) in (\"\")"=w168) -> ("States Out"=w169:string)  [unwired: 14 in]
          }
          event "Set_MWIR": Value Change {
            # "Go to state \"Hardware: Init EGSE\""
            n66 = event-data() -> ()  [unwired: 1 in, 6 out]
            n67 = Unbundle By Name(w175) -> ("MWIR CurrentSource"=w174:refnum<k24>)
            n68 = local read "Vout5_Res"() -> (w171:dbl)
            n69 = call "Set Current.vi"("Vout5_Res"=w171, "SWIR?"=FALSE, "Current"="MWIR Current", "task in"=w174) -> ()  [unwired: 6 in, 2 out]
            n70 = call <vilib>:"Add State(s) to Queue__jki_lib_state_machine.vi"("State(s) in (\"\")"=w176) -> ("States Out"=w177:string)  [unwired: 14 in]
          }
          event "Connect B2901BL": Value Change {
            # "Go to state \"Hardware: Init ISource or Hardware: Close ISource\""
            n71 = event-data() -> ()  [unwired: 1 in, 6 out]
            n72 = Unbundle By Name(w183) -> ("B2901 connected"=w182:bool)
            n73 = Select(t="Hardware: Close B2901", s=w182, f="Hardware: Init B2901" ("State(s) in Front (\"\")")) -> (s? t:f=w180:string)
            n74 = call <vilib>:"Add State(s) to Queue__jki_lib_state_machine.vi"("State(s) in Front (\"\")"=w180, "State(s) in (\"\")"=w184) -> ("States Out"=w185:string)  [unwired: 13 in]
          }
          event "Connect USB3104": Value Change {
            # "Go to state \"Hardware: Init ISource or Hardware: Close ISource\""
            n75 = event-data() -> ()  [unwired: 1 in, 6 out]
            n76 = Unbundle By Name(w191) -> ("USB3104 connected"=w190:bool)
            n77 = Select(t="Hardware: Close USB3104", s=w190, f="Hardware: Init USB3104" ("State(s) in Front (\"\")")) -> (s? t:f=w188:string)
            n78 = call <vilib>:"Add State(s) to Queue__jki_lib_state_machine.vi"("State(s) in Front (\"\")"=w188, "State(s) in (\"\")"=w192) -> ("States Out"=w193:string)  [unwired: 13 in]
          }
          event "Connect PicoAmmeter": Value Change {
            # "Go to state \"Hardware: Init ISource or Hardware: Close ISource\""
            n79 = event-data() -> ()  [unwired: 1 in, 6 out]
            n80 = Unbundle By Name(w199) -> ("Picoammeter connected"=w198:bool)
            n81 = Select(t="Hardware: Close PicoAmmeter", s=w198, f="Hardware: Init PicoAmmeter" ("State(s) in Front (\"\")")) -> (s? t:f=w196:string)
            n82 = call <vilib>:"Add State(s) to Queue__jki_lib_state_machine.vi"("State(s) in Front (\"\")"=w196, "State(s) in (\"\")"=w200) -> ("States Out"=w201:string)  [unwired: 13 in]
          }
          event "Find Offset": Value Change {
            n83 = event-data() -> ()  [unwired: 1 in, 6 out]
            n84 = Unbundle By Name(w204) -> ("Detector Resource"=w205:refnum<visa-resource-name>)
            n85 = property on="Finding Offset..." class="Bool (strict)"(error in=w208, "Value"=TRUE ("Searching...")) -> (error out=w213:errorcluster)  [unwired: 1 in, 1 out]
            n86 = while {
              shift-right: [w231] -> _
              shift-left: 4095 -> [w226]
              shift-right: [w230] -> _
              shift-left: 1 -> [w227]
              tunnel: w213 -> [w236]
              tunnel: [w222] -> w214
              tunnel: "Channel to Adjust" -> [w233]
              tunnel: w205 -> [w232]
              tunnel: [w229] -> w216 mode=indexing
              tunnel: [w228] -> w215 mode=indexing
              tunnel: [w221] -> w217 mode=indexing
              tunnel: [w224] -> w220 mode=indexing
              stop <- w237 stop-if-true
              n87 = Subtract(x=w226, y=w227) -> (x-y=w239:i32)
              n88 = Absolute Value(x=w239) -> (abs(x)=w235:i32)
              n89 = Less Or Equal?(x=w235, y=1) -> (x <= y?=w238:bool)
              n90 = case shown="False" w238 {
                tunnel: w226 -> [w253 w291]
                tunnel: w227 -> [w252 w293]
                tunnel: [w251 w293] -> w230
                tunnel: [w254 TRUE] -> w237
                tunnel: w236 -> [w265 _]
                tunnel: [w249 w291] -> w231
                tunnel: [w248 _] -> w223
                tunnel: w233 -> [w240 _]
                tunnel: w232 -> [w242 _]
                tunnel: [w243 w291] -> w225
                frame False {
                  w244 = 1 ("Avg")
                  # "Not there yet."
                  n91 = Add(x=w253, y=w252) -> (x+y=w267:i32)
                  n92 = Equal To 0?(x=w240) -> (x = 0?=w241:bool)
                  n93 = Quotient & Remainder(x=w267, y=2) -> (floor(x/y)=w243:i32)  [unwired: 1 out]
                  n94 = case shown="False" w241 {
                    tunnel: w243 -> [w268 w269]
                    frame False {
                      n95 = local write "MWIR DAC"(w268) -> ()
                    }
                    frame True {
                      n96 = local write "SWIR DAC"(w269) -> ()
                    }
                  }
                  n97 = call <instrlib>:"Set DAC.vi"("error in (no error)"=w265, "value (0)"=w243, "chan (0)"=w240, "VISA resource name"=w242) -> ("error out"=w264:errorcluster, "VISA resource name out"=w261:refnum<visa-resource-name>)  [unwired: 6 in]
                  n98 = call <userlib>:"Wait (ms)__ogtk.vi"("error in (no error)"=w264, "milliseconds to wait"=u32 5) -> ("error out"=w262:errorcluster)  [unwired: 8 in, 1 out]
                  n99 = local read "Oversample"() -> (w260:i32)
                  n100 = for {
                    N: w244 -> [_]
                    tunnel: w261 -> [w274]
                    tunnel: [w272] -> w259 mode=indexing
                    tunnel: w240 -> [w270]
                    shift-right: [w271] -> w248
                    shift-left: w262 -> [w275]
                    w273 = u16 0 items=["High", "Med", "Low"] ("Gain")
                    n101 = call <instrlib>:"Get ADC.vi"("Gain"=w273, "Detector"=w270, "error in (no error)"=w275, "VISA resource name"=w274) -> ("error out"=w271:errorcluster, "output"=w272:i32)  [unwired: 5 in, 1 out]
                  }
                  n102 = Add Array Elements(numeric array=w259) -> (sum=w246:i32)
                  n103 = Divide(x=w246, y=w244) -> (x/y=w245:dbl)
                  n104 = Divide(x=w245, y=w260) -> (x/y=w247:dbl)
                  n105 = Subtract(x=w247, y="Target Counts") -> (x-y=w250:dbl)
                  n106 = local write "Counts"(w247) -> ()
                  n107 = Absolute Value(x=w250) -> (abs(x)=w257:dbl)
                  n108 = Less?(x=w257, y="Tolerance") -> (x < y?=w255:bool)
                  n109 = case shown="False" w255 {
                    tunnel: [FALSE TRUE] -> w254
                    tunnel: w243 -> [w279 w289]
                    tunnel: w253 -> [w280 w288]
                    tunnel: w252 -> [w278 _]
                    tunnel: [w276 w289] -> w251
                    tunnel: w250 -> [w282 _]
                    tunnel: [w277 w288] -> w249
                    frame False {
                      # "Not there, so examine difference\nbetween target and reading"
                      n110 = Greater Than 0?(x=w282) -> (x > 0?=w281:bool)
                      n111 = case shown="False" w281 {
                        tunnel: w280 -> [_ w287]
                        tunnel: w279 -> [w285 w286]
                        tunnel: w278 -> [w284 _]
                        tunnel: [w285 w287] -> w277
                        tunnel: [w284 w286] -> w276
                        frame False {
                          # "Reading is below target, so next DAC vaue will be below midpoint"
                        }
                        frame True {
                          # "If reading is above target, then next DAC value will be above mid"
                        }
                      }
                    }
                    frame True {
                      # "Within tolerance, so finish"
                    }
                  }
                }
                frame True {
                  # "DAC Values identical so finish"
                }
              }
              n112 = property on="Counts" class="WFChart (strict)"(error in=w223) -> (error out=w222:errorcluster, "Value"=w221:dbl)  [unwired: 1 in, 1 out]
              n113 = To Double Precision Float(number=w226) -> (double precision float=w229:dbl)
              n114 = To Double Precision Float(number=w225) -> (double precision float=w224:dbl)
              n115 = To Double Precision Float(number=w227) -> (double precision float=w228:dbl)
            }
            n116 = Build Array(w215, w216, w220, w217) -> (w218:dbl[][])
            n117 = property on="Finding Offset..." class="Bool (strict)"(error in=w214, "Value"=FALSE ("Searching...")) -> (error out=w207:errorcluster)  [unwired: 1 in, 1 out]
            n118 = Transpose 2D Array(2D array=w218) -> (transposed array=→"Searching":dbl[][])
          }
          event "DecadeSweep": Value Change {
            n119 = event-data() -> ("NewVal"=w297:bool)  [unwired: 1 in, 5 out]
            n120 = case shown="False" w297 {
              frame True {
                w298 = T6."Enabled" ("Disabled")
                w299 = T6."Disabled and Grayed Out" ("Disabled")
                n121 = property on="MaxCurrent" class="DigNum (strict)"("DisabledEnum"=w299) -> ()  [unwired: 2 in, 2 out]
                n122 = property on="NPoints" class="DigNum (strict)"("DisabledEnum"=w299) -> ()  [unwired: 2 in, 2 out]
                n123 = property on="NPointsPerDecade" class="Ring (strict)"("DisabledEnum"=w298) -> ()  [unwired: 2 in, 2 out]
                n124 = property on="NumberDecades" class="DigNum (strict)"("DisabledEnum"=w298) -> ()  [unwired: 2 in, 2 out]
              }
              frame False {
                w300 = T6."Disabled and Grayed Out" ("Disabled")
                w301 = T6."Enabled" ("Disabled")
                n125 = property on="MaxCurrent" class="DigNum (strict)"("DisabledEnum"=w301) -> ()  [unwired: 2 in, 2 out]
                n126 = property on="NPoints" class="DigNum (strict)"("DisabledEnum"=w301) -> ()  [unwired: 2 in, 2 out]
                n127 = property on="NPointsPerDecade" class="Ring (strict)"("DisabledEnum"=w300) -> ()  [unwired: 2 in, 2 out]
                n128 = property on="NumberDecades" class="DigNum (strict)"("DisabledEnum"=w300) -> ()  [unwired: 2 in, 2 out]
              }
            }
          }
          event "SPI Clock": Value Change {
            # "SPI Clock changed"
            n129 = event-data() -> ()  [unwired: 1 in, 6 out]
            n130 = Unbundle By Name(w304) -> ("Detector Resource"=w305:refnum<visa-resource-name>)
            n131 = call <instrlib>:"Set Clock.vi"("error in (no error)"=w303, "ClockSpeed"="SPI Clock", "VISA resource name"=w305) -> ("error out"=w302:errorcluster)  [unwired: 7 in, 1 out]
          }
          event "Board Power": Value Change {
            # "Board Power changed"
            n132 = event-data() -> ()  [unwired: 1 in, 6 out]
            n133 = Unbundle By Name(w312) -> ("Detector Resource"=w308:refnum<visa-resource-name>)
            n134 = call <instrlib>:"Set Power.vi"("error in (no error)"=w309, "Power (0)"="Board Power", "VISA resource name"=w308) -> ("error out"=w310:errorcluster)  [unwired: 7 in, 1 out]
          }
          event "Heater Power": Value Change {
            # "Board Power changed"
            n135 = event-data() -> ()  [unwired: 1 in, 6 out]
            n136 = Unbundle By Name(w318) -> ("Detector Resource"=w314:refnum<visa-resource-name>)
            n137 = call <instrlib>:"Set Heater.vi"("error in (no error)"=w315, "Power (0)"="Heater Power", "VISA resource name"=w314) -> ("error out"=w316:errorcluster)  [unwired: 7 in, 1 out]
          }
          event "Manual LightSweep": Value Change {
            n138 = event-data() -> ()  [unwired: 1 in, 6 out]
            n139 = case shown="True" "Manual LightSweep" {
              tunnel: w322 -> [w325 w330]
              tunnel: [w325 w329] -> w321
              tunnel: w320 -> [_ w328]
              frame False {
              }
              frame True {
                w333 = dbl[] []
                n140 = Unbundle By Name(w328) -> ("Detector Resource"=w327:refnum<visa-resource-name>, "PicoAmmeter Resource"=w326:refnum<visa-resource-name>)
                n141 = local read "Oversample"() -> (w334:i32)
                n142 = while {
                  tunnel: [w365] -> w331
                  shift-right: [w368] -> _
                  shift-left: w333 -> [w370]
                  shift-right: [w358] -> _
                  shift-left: w333 -> [w360]
                  shift-right: [w357] -> _
                  shift-left: w333 -> [w359]
                  tunnel: "Detector 2" -> [w348]
                  tunnel: w327 -> [w347]
                  tunnel: w334 -> [w346]
                  shift-right: [w341] -> _
                  shift-left: w333 -> [w343]
                  tunnel: [w339] -> _
                  tunnel: w330 -> [w338]
                  tunnel: w326 -> [w336]
                  stop <- "StopGathering" stop-if-true
                  w361 = u16 2 items=["High", "Med", "Low"] ("Gain")
                  w362 = u16 1 items=["High", "Med", "Low"] ("Gain")
                  w371 = u16 0 items=["High", "Med", "Low"] ("Gain")
                  n143 = flat-sequence {
                    tunnel: w338 -> [w372]
                    tunnel: [w372] -> w337
                    frame #0 {
                      n144 = Wait Until Next ms Multiple(millisecond multiple="millisecond multiple") -> ()  [unwired: 1 out]
                    }
                  }
                  n145 = call <instrlib>:"Measure Current.vi"("VISA resource name"=w336, "error in (no error)"=w337) -> ("VISA resource name out"=w339:refnum<visa-resource-name>, "Measurement"=w342:dbl, "error out"=w344:errorcluster)  [unwired: 11 in]
                  "PhotoDiode" <- w342
                  n146 = Build Array (concatenate)(w343, w342) -> (w341:dbl[])
                  n147 = call <instrlib>:"Get ADC.vi"("Gain"=w371, "Detector"=w348, "error in (no error)"=w344, "VISA resource name"=w347) -> ("error out"=w367:errorcluster, "output"=w369:i32, "VISA resource name out"=w364:refnum<visa-resource-name>)  [unwired: 5 in]
                  n148 = Divide(x=w369, y=w346) -> (x/y=w349:dbl)
                  n149 = call <instrlib>:"Get ADC.vi"("Gain"=w362, "Detector"=w348, "error in (no error)"=w367, "VISA resource name"=w364) -> ("error out"=w366:errorcluster, "output"=w353:i32, "VISA resource name out"=w363:refnum<visa-resource-name>)  [unwired: 5 in]
                  n150 = Divide(x=w353, y=w346) -> (x/y=w350:dbl)
                  n151 = call <instrlib>:"Get ADC.vi"("Gain"=w361, "Detector"=w348, "error in (no error)"=w366, "VISA resource name"=w363) -> ("error out"=w365:errorcluster, "output"=w352:i32)  [unwired: 5 in, 1 out]
                  n152 = Divide(x=w352, y=w346) -> (x/y=w351:dbl)
                  n153 = Build Array (concatenate)(w360, w350) -> (w358:dbl[])
                  n154 = Build Array (concatenate)(w370, w349) -> (w368:dbl[])
                  n155 = Build Array (concatenate)(w359, w351) -> (w357:dbl[])
                  n156 = Bundle(w341, w368) -> (w356:cluster{dbl[], dbl[]})  [unwired: 1 in]
                  n157 = Bundle(w341, w358) -> (w355:cluster{dbl[], dbl[]})  [unwired: 1 in]
                  n158 = Bundle(w341, w357) -> (w354:cluster{dbl[], dbl[]})  [unwired: 1 in]
                  n159 = Build Array(w356, w355, w354) -> (→"Output vs Light 2":cluster{dbl[], dbl[]}[])
                }
                n160 = property on="StopGathering" class="Bool (strict)"(error in=w331, "Value"=FALSE ("StopGathering")) -> (error out=w329:errorcluster)  [unwired: 1 in, 1 out]
              }
            }
          }
          event "SweepVDAC": Value Change {
            n161 = event-data() -> ()  [unwired: 1 in, 6 out]
            n162 = case shown="True" "SweepVDAC" {
              tunnel: w376 -> [w379 w383]
              tunnel: [w379 w382] -> w375
              tunnel: w374 -> [_ w380]
              frame False {
              }
              frame True {
                w391 = dbl[] []
                n163 = Unbundle By Name(w380) -> ("Detector Resource"=w381:refnum<visa-resource-name>)
                n164 = call-poly <vilib>:"Ramp Pattern.vi"("start"="VDAC Min", "end"="VDAC Max", "delta"="VDAC Step") -> ("Ramp Pattern"=w392:dbl[])  [unwired: 6 in, 2 out]
                n165 = local read "Oversample"() -> (w390:i32)
                n166 = for {
                  tunnel: w392 -> [w411] mode=indexing
                  tunnel: [w407] -> w382
                  shift-right: [w408] -> _
                  shift-left: w391 -> [w409]
                  tunnel: w392 -> [w402]
                  tunnel: w381 -> [w398]
                  shift-right: [w404] -> _
                  shift-left: w391 -> [w406]
                  shift-right: [w403] -> _
                  shift-left: w391 -> [w405]
                  tunnel: w390 -> [w400]
                  tunnel: "Channel to Sweep" -> [w399]
                  tunnel: "Tab Control 2" -> [w396]
                  shift-right: [w394] -> _
                  shift-left: dbl[][] [] -> [w395]
                  tunnel: w383 -> [w393]
                  stop <- "Abort SweepVDAC" stop-if-true
                  n167 = call <instrlib>:"Set DAC.vi"("error in (no error)"=w393, "value (0)"=w411, "chan (0)"=w399, "VISA resource name"=w398) -> ("error out"=w410:errorcluster, "VISA resource name out"=w397:refnum<visa-resource-name>)  [unwired: 6 in]
                  n168 = case shown="\"Science Mode\"" w396 {
                    tunnel: w410 -> [w441 w453]
                    tunnel: w409 -> [w439 w451]
                    tunnel: [w437 w451] -> w408
                    tunnel: [w434 w452] -> w407
                    tunnel: w406 -> [w429 w450]
                    tunnel: w405 -> [w428 w449]
                    tunnel: [w427 w450] -> w404
                    tunnel: [w426 w449] -> w403
                    tunnel: w402 -> [w425 w446]
                    tunnel: w400 -> [w419 w442]
                    tunnel: w399 -> [w417 _]
                    tunnel: w397 -> [w416 w454]
                    tunnel: w395 -> [w412 w448]
                    tunnel: [w412 w444] -> w394
                    frame "Individual", Default {
                      w430 = u16 2 items=["High", "Med", "Low"] ("Gain")
                      w431 = u16 1 items=["High", "Med", "Low"] ("Gain")
                      w440 = u16 0 items=["High", "Med", "Low"] ("Gain")
                      n169 = call <instrlib>:"Get ADC.vi"("Gain"=w440, "Detector"=w417, "error in (no error)"=w441, "VISA resource name"=w416) -> ("error out"=w436:errorcluster, "output"=w438:i32, "VISA resource name out"=w433:refnum<visa-resource-name>)  [unwired: 5 in]
                      n170 = Divide(x=w438, y=w419) -> (x/y=w413:dbl)
                      n171 = call <instrlib>:"Get ADC.vi"("Gain"=w431, "Detector"=w417, "error in (no error)"=w436, "VISA resource name"=w433) -> ("error out"=w435:errorcluster, "output"=w420:i32, "VISA resource name out"=w432:refnum<visa-resource-name>)  [unwired: 5 in]
                      n172 = Divide(x=w420, y=w419) -> (x/y=w414:dbl)
                      n173 = call <instrlib>:"Get ADC.vi"("Gain"=w430, "Detector"=w417, "error in (no error)"=w435, "VISA resource name"=w432) -> ("error out"=w434:errorcluster, "output"=w418:i32)  [unwired: 5 in, 1 out]
                      n174 = Divide(x=w418, y=w419) -> (x/y=w415:dbl)
                      n175 = Build Array (concatenate)(w429, w414) -> (w427:dbl[])
                      n176 = Build Array (concatenate)(w439, w413) -> (w437:dbl[])
                      n177 = Build Array (concatenate)(w428, w415) -> (w426:dbl[])
                      n178 = Bundle("Ramp Pattern"=w425, w437) -> (w424:cluster{"Ramp Pattern":dbl[], dbl[]})  [unwired: 1 in]
                      n179 = Bundle("Ramp Pattern"=w425, w427) -> (w423:cluster{"Ramp Pattern":dbl[], dbl[]})  [unwired: 1 in]
                      n180 = Bundle("Ramp Pattern"=w425, w426) -> (w422:cluster{"Ramp Pattern":dbl[], dbl[]})  [unwired: 1 in]
                      n181 = Build Array(w424, w423, w422) -> (→"VDAC Sweep":cluster{"Ramp Pattern":dbl[], dbl[]}[])
                    }
                    frame "Science Mode" {
                      n182 = call <instrlib>:"Get SCIENCE.vi"("error in (no error)"=w453, "VISA resource name"=w454) -> ("error out"=w452:errorcluster, "subarray"=w445:dbl[])  [unwired: 6 in, 2 out]
                      n183 = Divide(x=w445, y=w442) -> (x/y=w443:dbl[])
                      n184 = Build Array (concatenate)(w448, w443) -> (w444:dbl[][])
                      n185 = call "Make Graph.vi"("SciData"=w444, "X-Data"=w446) -> ("All Counts 2"=→"Count cs DAC":cluster{"X-Data":dbl[], "SciData":dbl[]}[])  [unwired: 9 in]
                    }
                  }
                }
              }
            }
          }
          event "SWIR DAC": Value Change {
            w459 = 0  # chan (0)
            n186 = event-data() -> ()  [unwired: 1 in, 6 out]
            n187 = Unbundle By Name(w456) -> ("Detector Resource"=w455:refnum<visa-resource-name>)
            n188 = call <instrlib>:"Set DAC.vi"("value (0)"="SWIR DAC", "chan (0)"=w459, "VISA resource name"=w455) -> ()  [unwired: 7 in, 2 out]
          }
          event "MWIR DAC": Value Change {
            w465 = 1  # chan (0)
            n189 = event-data() -> ()  [unwired: 1 in, 6 out]
            n190 = Unbundle By Name(w462) -> ("Detector Resource"=w461:refnum<visa-resource-name>)
            n191 = call <instrlib>:"Set DAC.vi"("value (0)"="MWIR DAC", "chan (0)"=w465, "VISA resource name"=w461) -> ()  [unwired: 7 in, 2 out]
          }
          event "ResetVDACstats": Value Change {
            w467 = dbl[] [] ("History Data")
            n192 = event-data() -> ()  [unwired: 1 in, 6 out]
            n193 = property on="Counts" class="WFChart (strict)"("History Data"=w467) -> ()  [unwired: 2 in, 2 out]
            n194 = property on="Board RTD Value Temperature" class="WFChart (strict)"("History Data"=w467) -> ()  [unwired: 2 in, 2 out]
          }
          event "ResetScienceGraph": Value Change {
            n195 = event-data() -> ()  [unwired: 1 in, 6 out]
            n196 = property on="All Counts" class="WFChart (strict)"("History Data"=T3 []) -> ()  [unwired: 2 in, 2 out]
          }
          event "Export to Excel": Value Change {
            n197 = event-data() -> ()  [unwired: 1 in, 6 out]
            n198 = Empty String/Path?(string/path="test Results save directory") -> (empty?=w475:bool)
            n199 = case shown="False" w475 {
              tunnel: w478 -> [w483 w503]
              tunnel: [w482 w503] -> w477
              tunnel: "test Results save directory" -> [w481 _]
              frame False {
                w486 = "," ("delimiter (\\t)")
                n200 = Get Date/Time In Seconds() -> (seconds since 1Jan1904=w494:timestamp)
                n201 = Format Date/Time String(time format string (%c)="%Y%m%dT%H%M%S.csv", seconds (now)=w494) -> (date/time string=w495:string)  [unwired: 1 in]
                "Save FileName" <- w495
                n202 = Build Path(base path=w481, name or relative path=w495) -> (appended path=w496:path)
                n203 = for {
                  N: 10 -> [_]
                  tunnel: [w499] -> w492 mode=indexing
                  i -> [w501]
                  n204 = property on="All Counts" class="WFChart (strict)"("Active Plot"=w501) -> (error out=w500:errorcluster)  [unwired: 2 in, 1 out]
                  n205 = property on="All Counts" class="WFChart (strict)"(error in=w500) -> ("Plot.Plot Name"=w499:string)  [unwired: 1 in, 2 out]
                }
                n206 = property on="All Counts" class="WFChart (strict)"() -> ("History Data"=w493:T3)  [unwired: 2 in, 2 out]
                n207 = for {
                  tunnel: w493 -> [w498] mode=indexing
                  tunnel: [w497] -> w490 mode=indexing
                  n208 = Cluster To Array(cluster=w498) -> (array=w497:dbl[])
                }
                n209 = call-poly <vilib>:"Write Delimited Spreadsheet.vi"("file path (dialog if empty)"=w496, "1D data"=w492, "error in (no error)"=w483, "delimiter (\\t)"=w486) -> ("new file path (Not A Path if cancelled)"=w491:path, "error out"=w484:errorcluster)  [unwired: 10 in]
                n210 = call-poly <vilib>:"Write Delimited Spreadsheet.vi"("file path (dialog if empty)"=w491, "format (%.3f)"="%.4g", "2D data"=w490, "append to file? (new file:F)"=TRUE, "error in (no error)"=w484, "delimiter (\\t)"=w486) -> ("error out"=w482:errorcluster)  [unwired: 8 in, 1 out]
              }
              frame True {
                n211 = One Button Dialog(message="Results save directory cannot be empty\n\nPlease select a directory to store results in" ("source")) -> ()  [unwired: 1 in, 1 out]
              }
            }
          }
          event "Oversample": Value Change {
            n212 = event-data() -> ()  [unwired: 1 in, 6 out]
            n213 = Unbundle By Name(w505) -> ("Detector Resource"=w504:refnum<visa-resource-name>)
            n214 = call <instrlib>:"Set OverSample.vi"("oversample (0)"="Oversample", "VISA resource name"=w504) -> ()  [unwired: 8 in, 2 out]
          }
          event "B2901 Sweep": Value Change {
            n215 = event-data() -> ()  [unwired: 1 in, 6 out]
            n216 = Unbundle By Name(w510) -> ("PicoAmmeter Resource"=w512:refnum<visa-resource-name>, "Picoammeter connected"=w511:bool, "Detector Resource"=w517:refnum<visa-resource-name>, "B2901 connected"=w514:bool, "B2901 Resource"=w513:refnum<visa-resource-name>)
            n217 = case shown="True" w514 {
              tunnel: w517 -> [_ w532]
              tunnel: w516 -> [w520 w531]
              tunnel: [w520 w529] -> w515
              tunnel: w513 -> [_ w530]
              tunnel: w512 -> [_ w528]
              tunnel: w511 -> [_ w527]
              tunnel: w510 -> [w519 w523]
              tunnel: [w519 w522] -> w509
              frame False {
              }
              frame True {
                w541 = u16 1 items=["Voltage", "Current"] ("Source Mode  (0: Voltage)")
                w548 = u16 1 items=["Voltage", "Current"] ("Source Mode  (0: Voltage)")
                n218 = call <instrlib>:"Configure Output.vi"("Source Mode  (0: Voltage)"=w548, "error in (no error)"=w531, "Output Level (0)"=0.0, "VISA resource name"=w530) -> ("error out"=w547:errorcluster, "VISA resource name out"=w546:refnum<visa-resource-name>)  [unwired: 6 in]
                n219 = call <instrlib>:"Enable Output.vi"("error in (no error)"=w547, "Enable Output (T: Enable)"=TRUE ("Auto Output-Off (F: Disable)"), "VISA resource name"=w546) -> ("error out"=w544:errorcluster, "VISA resource name out"=w543:refnum<visa-resource-name>)  [unwired: 7 in]
                n220 = case shown="True" "DecadeSweep" {
                  tunnel: "MaxCurrent" -> [w557 _]
                  tunnel: "MinCurrent" -> [w556 w561]
                  tunnel: [w558 w560] -> w535
                  tunnel: "NumberDecades" -> [_ w562]
                  tunnel: "NPoints" -> [w555 _]
                  tunnel: "NPointsPerDecade" -> [_ w559]
                  frame False {
                    n221 = call-poly <vilib>:"Ramp Pattern.vi"("start"=w556, "end"=w557, "samples"=w555) -> ("Ramp Pattern"=w558:dbl[])  [unwired: 7 in, 1 out]
                  }
                  frame True {
                    n222 = call "Decades125.vi"("NPointsPerDecade"=w559, "BaseUnit"=w561, "NumberDecades"=w562) -> ("output array"=w560:dbl[])  [unwired: 8 in]
                  }
                }
                n223 = call <userlib>:"Wait (ms)__ogtk.vi"("error in (no error)"=w544, "milliseconds to wait"=u32 1000) -> ("error out"=w551:errorcluster)  [unwired: 8 in, 1 out]
                n224 = local read "Oversample"() -> (w553:i32)
                n225 = for {
                  tunnel: w551 -> [w586]
                  tunnel: w535 -> [w582] mode=indexing
                  tunnel: [w567] -> w536
                  shift-right: [w573] -> _
                  shift-left: dbl[][] [] -> [w587]
                  tunnel: w535 -> [w574]
                  tunnel: w532 -> [w577]
                  tunnel: w553 -> [w571]
                  tunnel: [w585] -> w537
                  tunnel: w543 -> [w580]
                  tunnel: w528 -> [w565]
                  tunnel: w527 -> [w564]
                  tunnel: [w563] -> w521
                  w581 = u16 1 items=["Voltage", "Current"] ("Source Mode  (0: Voltage)")
                  n226 = call <instrlib>:"Configure Output.vi"("Source Mode  (0: Voltage)"=w581, "error in (no error)"=w586, "Output Level (0)"=w582, "VISA resource name"=w580) -> ("error out"=w584:errorcluster, "VISA resource name out"=w585:refnum<visa-resource-name>)  [unwired: 6 in]
                  n227 = call <userlib>:"Wait Until Next ms Multiple__ogtk.vi"("error in (no error)"=w584, "milliseconds to wait"=u32 100) -> ("error out"=w576:errorcluster)  [unwired: 8 in, 1 out]
                  n228 = call <instrlib>:"Get SCIENCE.vi"("error in (no error)"=w576, "VISA resource name"=w577) -> ("error out"=w579:errorcluster, "subarray"=w575:dbl[], "VISA resource name out"=w578:refnum<visa-resource-name>)  [unwired: 6 in, 1 out]
                  n229 = Divide(x=w575, y=w571) -> (x/y=w572:dbl[])
                  n230 = call "Get Temperature.vi"("error in (no error)"=w579, "VISA resource name"=w578) -> ("error out"=w568:errorcluster, "output"=w569:dbl)  [unwired: 7 in, 1 out]
                  n231 = call "ReadPicoAmmeter.vi"("error in (no error)"=w568, "Connected"=w564, "PicoAmmeter"=w565) -> ("error out"=w567:errorcluster, "Current"=w566:dbl)  [unwired: 7 in]
                  n232 = Build Array (concatenate)(w572, w569, w566) -> (w570:dbl[])
                  n233 = Build Array (concatenate)(w587, w570) -> (w573:dbl[][])
                  n234 = call "Make Graph.vi"("SciData"=w573, "X-Data"=w574) -> ("All Counts 2"=w563:cluster{"X-Data":dbl[], "SciData":dbl[]}[])  [unwired: 9 in]
                  "OutputCurrentGrph" <- w563
                }
                n235 = Bundle By Name(cluster=w523, "OpVsCurrent"=w521) -> (w522:T8)
                n236 = call <instrlib>:"Configure Output.vi"("Source Mode  (0: Voltage)"=w541, "error in (no error)"=w536, "Output Level (0)"=0.0, "VISA resource name"=w537) -> ("error out"=w539:errorcluster, "VISA resource name out"=w538:refnum<visa-resource-name>)  [unwired: 6 in]
                n237 = call <instrlib>:"Enable Output.vi"("error in (no error)"=w539, "Enable Output (T: Enable)"=FALSE ("Auto Output-Off (F: Disable)"), "VISA resource name"=w538) -> ("error out"=w529:errorcluster)  [unwired: 7 in, 1 out]
              }
            }
          }
          event "SWIR sweep USB3104", "MWIR sweep USB3104": Value Change {
            n238 = event-data() -> ()  [unwired: 1 in, 6 out]
            n239 = Unbundle By Name(w592) -> ("PicoAmmeter Resource"=w597:refnum<visa-resource-name>, "Picoammeter connected"=w596:bool, "Detector Resource"=w601:refnum<visa-resource-name>, "USB3104 connected"=w598:bool, "Vout5_Res"=w589:dbl, "Vout3_Res"=w588:dbl, "SWIR CurrentSource"=w590:refnum<k24>, "MWIR CurrentSource"=w595:refnum<k24>)
            n240 = Select(t=w590, s="SWIR sweep USB3104", f=w595) -> (s? t:f=w594:refnum<k24>)
            n241 = case shown="True" w598 {
              tunnel: w601 -> [_ w632]
              tunnel: w600 -> [w604 w623]
              tunnel: [w604 w616] -> w599
              tunnel: w597 -> [_ w631]
              tunnel: w596 -> [_ w630]
              tunnel: w594 -> [_ w621]
              tunnel: "SWIR sweep USB3104" -> [_ w618]
              tunnel: w592 -> [w603 w612]
              tunnel: [w603 w611] -> w591
              tunnel: w589 -> [_ w608]
              tunnel: w588 -> [_ w607]
              frame False {
              }
              frame True {
                n242 = local read "NumberDecades"() -> (w626:i32)
                n243 = local read "DecadeSweep"() -> (w624:bool)
                n244 = local read "MaxCurrent"() -> (w627:dbl)
                n245 = local read "MinCurrent"() -> (w625:dbl)
                n246 = local read "NPointsPerDecade"() -> (w605:u16)
                n247 = local read "NPoints"() -> (w628:i32)
                n248 = call "Set Current.vi"("Vout5_Res"=w608, "SWIR?"=w618, "Vout3_Res"=w607, "error in (no error)"=w623, "Current"=0.0, "task in"=w621) -> ("error out"=w622:errorcluster, "task out"=w619:refnum<k24>)  [unwired: 4 in]
                n249 = case shown="True" w624 {
                  tunnel: w627 -> [w638 _]
                  tunnel: w625 -> [w637 w642]
                  tunnel: [w639 w641] -> w633
                  tunnel: w626 -> [_ w643]
                  tunnel: w628 -> [w636 _]
                  tunnel: w605 -> [_ w640]
                  frame False {
                    n250 = call-poly <vilib>:"Ramp Pattern.vi"("start"=w637, "end"=w638, "samples"=w636) -> ("Ramp Pattern"=w639:dbl[])  [unwired: 7 in, 1 out]
                  }
                  frame True {
                    n251 = call "Decades125.vi"("NPointsPerDecade"=w640, "BaseUnit"=w642, "NumberDecades"=w643) -> ("output array"=w641:dbl[])  [unwired: 8 in]
                  }
                }
                n252 = call <userlib>:"Wait (ms)__ogtk.vi"("error in (no error)"=w622, "milliseconds to wait"=u32 1000) -> ("error out"=w635:errorcluster)  [unwired: 8 in, 1 out]
                n253 = for {
                  tunnel: w635 -> [w669]
                  tunnel: w633 -> [w665] mode=indexing
                  tunnel: [w652] -> w617
                  shift-right: [w657] -> _
                  shift-left: dbl[][] [] -> [w670]
                  tunnel: w633 -> [w658]
                  tunnel: w632 -> [w661]
                  tunnel: [w668] -> w614
                  tunnel: w619 -> [w664]
                  tunnel: w631 -> [w650]
                  tunnel: w630 -> [w649]
                  tunnel: [w648] -> w610
                  tunnel: w618 -> [w646]
                  tunnel: [w646] -> w613
                  tunnel: [w645] -> w609
                  tunnel: w608 -> [w645]
                  tunnel: w607 -> [w644]
                  tunnel: [w644] -> w606
                  n254 = call "Set Current.vi"("Vout5_Res"=w645, "SWIR?"=w646, "Vout3_Res"=w644, "error in (no error)"=w669, "Current"=w665, "task in"=w664) -> ("error out"=w667:errorcluster, "task out"=w668:refnum<k24>)  [unwired: 4 in]
                  n255 = local read "Oversample"() -> (w647:i32)
                  n256 = call <userlib>:"Wait Until Next ms Multiple__ogtk.vi"("error in (no error)"=w667, "milliseconds to wait"=u32 100) -> ("error out"=w660:errorcluster)  [unwired: 8 in, 1 out]
                  n257 = call <instrlib>:"Get SCIENCE.vi"("error in (no error)"=w660, "VISA resource name"=w661) -> ("error out"=w663:errorcluster, "subarray"=w659:dbl[], "VISA resource name out"=w662:refnum<visa-resource-name>)  [unwired: 6 in, 1 out]
                  n258 = Divide(x=w659, y=w647) -> (x/y=w656:dbl[])
                  n259 = call "Get Temperature.vi"("error in (no error)"=w663, "VISA resource name"=w662) -> ("error out"=w653:errorcluster, "output"=w654:dbl)  [unwired: 7 in, 1 out]
                  n260 = call "ReadPicoAmmeter.vi"("error in (no error)"=w653, "Connected"=w649, "PicoAmmeter"=w650) -> ("error out"=w652:errorcluster, "Current"=w651:dbl)  [unwired: 7 in]
                  n261 = Build Array (concatenate)(w656, w654, w651) -> (w655:dbl[])
                  n262 = Build Array (concatenate)(w670, w655) -> (w657:dbl[][])
                  n263 = call "Make Graph.vi"("SciData"=w657, "X-Data"=w658) -> ("All Counts 2"=w648:cluster{"X-Data":dbl[], "SciData":dbl[]}[])  [unwired: 9 in]
                  n264 = local write "OutputCurrentGrph"(w648) -> ()
                }
                n265 = Bundle By Name(cluster=w612, "OpVsCurrent"=w610) -> (w611:T8)
                n266 = call "Set Current.vi"("Vout5_Res"=w609, "SWIR?"=w613, "Vout3_Res"=w606, "error in (no error)"=w617, "Current"=0.0, "task in"=w614) -> ("error out"=w616:errorcluster)  [unwired: 4 in, 1 out]
              }
            }
          }
          event "Vout5 Sweep", "Vout3 Sweep": Value Change {
            n267 = event-data() -> ()  [unwired: 1 in, 6 out]
            n268 = Unbundle By Name(w673) -> ("PicoAmmeter Resource"=w678:refnum<visa-resource-name>, "Picoammeter connected"=w677:bool, "USB3104 connected"=w679:bool, "SWIR CurrentSource"=w676:refnum<k24>, "MWIR CurrentSource"=w675:refnum<k24>)
            n269 = Select(t=w676, s="Vout3 Sweep", f=w675) -> (s? t:f=w674:refnum<k24>)
            n270 = case shown="True" w679 {
              tunnel: w681 -> [w684 w712]
              tunnel: [w684 w707] -> w680
              tunnel: w678 -> [_ w714]
              tunnel: w677 -> [_ w713]
              tunnel: w674 -> [_ w710]
              tunnel: w673 -> [w683 w687]
              tunnel: [w683 w686] -> w672
              tunnel: "Vout3 Sweep" -> [_ w688]
              frame False {
              }
              frame True {
                n271 = call <instrlib>:"ULx Write (Analog 1D DBL 1Chan 1Samp).vi"("task in"=w710, "data"=0.0 ("Current"), "error in"=w712) -> ("task out"=w709:refnum<k24>, "error out"=w711:errorcluster)  [unwired: 10 in, 1 out]
                n272 = Increment(x="NPoints 2") -> (x+1=w697:i32)
                n273 = Select(t="Vout3" ("T button name (\"OK\")"), s=w688, f="Vout5" ("T button name (\"OK\")")) -> (s? t:f=w693:string)
                n274 = call <userlib>:"Wait (ms)__ogtk.vi"("error in (no error)"=w711, "milliseconds to wait"=u32 1000) -> ("error out"=w717:errorcluster)  [unwired: 8 in, 1 out]
                n275 = call-poly <vilib>:"Ramp Pattern.vi"("start"="MinVoltage", "end"="MaxVoltage", "samples"=w697) -> ("Ramp Pattern"=w715:dbl[])  [unwired: 7 in, 1 out]
                n276 = for {
                  tunnel: w717 -> [w742]
                  tunnel: w715 -> [w732] mode=indexing
                  tunnel: [w736] -> w708
                  shift-right: [w729] -> _
                  shift-left: dbl[] [] -> [w743]
                  tunnel: w715 -> [w730]
                  tunnel: [w741] -> w706
                  tunnel: w709 -> [w738]
                  tunnel: w714 -> [w734]
                  tunnel: w713 -> [w733]
                  tunnel: [w730] -> w700
                  tunnel: [w729] -> w699
                  n277 = call <instrlib>:"ULx Write (Analog 1D DBL 1Chan 1Samp).vi"("task in"=w738, "data"=w732, "error in"=w742) -> ("task out"=w741:refnum<k24>, "error out"=w740:errorcluster)  [unwired: 10 in, 1 out]
                  n278 = call <userlib>:"Wait Until Next ms Multiple__ogtk.vi"("error in (no error)"=w740, "milliseconds to wait"=u32 100) -> ("error out"=w737:errorcluster)  [unwired: 8 in, 1 out]
                  n279 = call "ReadPicoAmmeter.vi"("error in (no error)"=w737, "Connected"=w733, "PicoAmmeter"=w734) -> ("error out"=w736:errorcluster, "Current"=w735:dbl)  [unwired: 7 in]
                  n280 = Build Array (concatenate)(w743, w735) -> (w729:dbl[])
                  n281 = Bundle("Ramp Pattern"=w730, w729) -> (→"IV Graph":cluster{"Ramp Pattern":dbl[], dbl[]})  [unwired: 1 in]
                }
                n282 = call <vilib>:"Linear Fit.vi"("Y"=w700, "X"=w699) -> ("slope"=w685:dbl)  [unwired: 9 in, 4 out]
                "Resistance (Ohms)" <- w685
                n283 = call <instrlib>:"ULx Write (Analog 1D DBL 1Chan 1Samp).vi"("task in"=w706, "data"=0.0 ("Current"), "error in"=w708) -> ("error out"=w707:errorcluster)  [unwired: 10 in, 2 out]
                n284 = Format Into String(format string="Resistor value  of %g found for %s channel\\nTransfer to current source data?" ("message"), w685, w693) -> (resulting string=w692:string)  [unwired: 2 in, 1 out]
                n285 = Two Button Dialog(message=w692, 1:"No" ("F button name (\"Cancel\")"), 2:"Yes" ("T button name (\"OK\")")) -> (T button?=w689:bool)
                n286 = case shown="True" w689 {
                  tunnel: w688 -> [_ w722]
                  tunnel: w687 -> [w718 w721]
                  tunnel: [w718 w720] -> w686
                  tunnel: w685 -> [_ w719]
                  frame False {
                  }
                  frame True {
                    n287 = case shown="False" w722 {
                      tunnel: w721 -> [w725 w728]
                      tunnel: [w724 w727] -> w720
                      tunnel: w719 -> [w723 w726]
                      frame True {
                        n288 = Bundle By Name(cluster=w725, "Vout3_Res"=w723) -> (w724:T8)
                        n289 = local write "Vout3_Res"(w723) -> ()
                      }
                      frame False {
                        n290 = local write "Vout5_Res"(w726) -> ()
                        n291 = Bundle By Name(cluster=w728, "Vout5_Res"=w726) -> (w727:T8)
                      }
                    }
                  }
                }
              }
            }
          }
          event "ThrowAway": Value Change {
            n292 = event-data() -> ()  [unwired: 1 in, 6 out]
            n293 = Unbundle By Name(w746) -> ("Detector Resource"=w744:refnum<visa-resource-name>)
            n294 = call <instrlib>:"Set ThrowAway.vi"("ThrowAway (0)"="ThrowAway", "VISA resource name"=w744) -> ()  [unwired: 8 in, 2 out]
          }
          event "OutputCurrentGrph": Cursor Release {
            w755 = T9 0 items=["Least Square", "Least Absolute Residual", "Bisquare"] ("method")
            n295 = event-data() -> ()  [unwired: 1 in, 9 out]
            n296 = Unbundle By Name(w750) -> ("OpVsCurrent"=w749:cluster{"Ramp Pattern":dbl[], dbl[]}[])
            n297 = property on="OutputCurrentGrph" class="XYGraph (strict)"("Active Cursor"=u32 0) -> (error out=w757:errorcluster)  [unwired: 2 in, 1 out]
            n298 = property on="OutputCurrentGrph" class="XYGraph (strict)"(error in=w757) -> (error out=w759:errorcluster, "Cursor.Cursor Position"=w760:T10)  [unwired: 1 in, 1 out]
            n299 = Unbundle By Name(w760) -> ("Cursor X"=w771:dbl)
            n300 = property on="OutputCurrentGrph" class="XYGraph (strict)"(error in=w759, "Active Cursor"=u32 1) -> (error out=w758:errorcluster)  [unwired: 1 in, 1 out]
            n301 = property on="OutputCurrentGrph" class="XYGraph (strict)"(error in=w758) -> ("Cursor.Cursor Position"=w761:T10)  [unwired: 1 in, 2 out]
            n302 = Index Array(array=w749) -> (element=w774:cluster{"Ramp Pattern":dbl[], dbl[]})  [unwired: 1 in]
            n303 = Unbundle(w774) -> ("Ramp Pattern"=w762:dbl[], w764:dbl[])
            n304 = Unbundle By Name(w761) -> ("Cursor X"=w770:dbl)
            n305 = Max & Min(x=w770, y=w771) -> (max(x,y)=w773:dbl, min(x,y)=w772:dbl)
            n306 = Search 1D Array(1D array=w762, element=w772) -> (index of element=w765:i32)  [unwired: 1 in]
            n307 = Search 1D Array(1D array=w762, element=w773) -> (index of element=w763:i32)  [unwired: 1 in]
            n308 = Subtract(x=w763, y=w765) -> (x-y=w766:i32)
            n309 = Array Subset(array=w764, index=w765, length=w766) -> (w780:dbl[])
            n310 = Array Subset(array=w762, index=w765, length=w766) -> (w775:dbl[])
            n311 = call <vilib>:"Linear Fit.vi"("Y"=w780, "X"=w775, "method"=w755) -> ("Best Linear Fit"=w779:dbl[], "slope"=→"slope (counts/nA)":dbl, "intercept"=→"intercept":dbl, "residue"=→"residue":dbl)  [unwired: 8 in, 1 out]
            n312 = Bundle(w775, "Best Linear Fit"=w779) -> (w777:cluster{dbl[], "Best Linear Fit":dbl[]})  [unwired: 1 in]
            n313 = Subtract(x=w780, y=w779) -> (x-y=w781:dbl[])
            n314 = local read "OutputCurrentGrph"() -> (w776:cluster{"Ramp Pattern":dbl[], dbl[]}[])
            n315 = Absolute Value(x=w781) -> (abs(x)=w782:dbl[])
            n316 = Array Max & Min(array=w782) -> (max value=→"Max Deviation (counts)":dbl)  [unwired: 3 out]
            n317 = Replace Array Subset(array=w776, new element=w777, index=1) -> (w778:cluster{"Ramp Pattern":dbl[], dbl[]}[])
            n318 = local write "OutputCurrentGrph"(w778) -> ()
          }
          event "SweepLight": Value Change {
            n319 = event-data() -> ()  [unwired: 1 in, 6 out]
            n320 = Unbundle By Name(w787) -> ("Detector Resource"=w786:refnum<visa-resource-name>)
            n321 = case shown="True" "SweepLight" {
              tunnel: w786 -> [_ w793]
              tunnel: w785 -> [w790 w792]
              tunnel: [w790 w791] -> w784
              frame False {
              }
              frame True {
                w810 = dbl[] []
                n322 = disable-structure shown="Disabled" {
                  disable-tunnel: [w819 _] -> w811
                  frame Disabled {
                    n323 = call "Keithley 648X Series SetupAcquisition.vi"("VISA resource name"=refnum<visa-resource-name> "Picoammeter") -> ("VISA resource name out"=w819:refnum<visa-resource-name>)  [unwired: 8 in, 1 out]
                  }
                  frame Enabled {
                  }
                }
                n324 = local read "Oversample"() -> (w818:i32)
                n325 = call-poly <vilib>:"Ramp Pattern.vi"("start"="Modulation Min", "end"="Modulation Max", "samples"="Modulation Steps") -> ("Ramp Pattern"=w814:dbl[])  [unwired: 7 in, 1 out]
                n326 = call <instrlib>:"Set DAC.vi"("error in (no error)"=w792, "value (0)"="DAC", "chan (0)"="Detector 7", "VISA resource name"=w793) -> ("error out"=w809:errorcluster, "VISA resource name out"=w817:refnum<visa-resource-name>)  [unwired: 6 in]
                n327 = call <instrlib>:"ULx Create Channel (AO-Voltage-Basic).vi"("maximum value"=5.0, "minimum value"=0.0, "physical channels"=refnum<k21> "Dev0/Ao0", "error in"=w809) -> ("task out"=w804:refnum<k24>, "error out"=w803:errorcluster)  [unwired: 10 in]
                n328 = call <instrlib>:"ULx Write (Analog 1D DBL 1Chan 1Samp).vi"("task in"=w804, "data"="Modulation Min", "error in"=w803) -> ("task out"=w805:refnum<k24>, "error out"=w800:errorcluster)  [unwired: 10 in, 1 out]
                n329 = call <userlib>:"Wait (ms)__ogtk.vi"("error in (no error)"=w800, "milliseconds to wait"=u32 1000) -> ("error out"=w801:errorcluster)  [unwired: 8 in, 1 out]
                n330 = for {
                  tunnel: w801 -> [w849]
                  tunnel: [w848] -> w795
                  tunnel: [w830] -> w797
                  shift-right: [w843] -> _
                  shift-left: w810 -> [w845]
                  tunnel: w817 -> [w842]
                  shift-right: [w838] -> _
                  shift-left: w810 -> [w840]
                  shift-right: [w837] -> _
                  shift-left: w810 -> [w839]
                  tunnel: w818 -> [w832]
                  tunnel: "Detector 7" -> [w831]
                  tunnel: w814 -> [w823] mode=indexing
                  tunnel: w811 -> [w829]
                  shift-right: [w825] -> _
                  shift-left: w810 -> [w826]
                  tunnel: w805 -> [w824]
                  stop <- "Abort 2" stop-if-true
                  n331 = call <instrlib>:"ULx Write (Analog 1D DBL 1Chan 1Samp).vi"("task in"=w824, "data"=w823, "error in"=w849) -> ("task out"=w848:refnum<k24>, "error out"=w847:errorcluster)  [unwired: 10 in, 1 out]
                  n332 = call <instrlib>:"Get ADC.vi"("Gain"="Gain 2", "Detector"=w831, "error in (no error)"=w847, "VISA resource name"=w842) -> ("error out"=w841:errorcluster, "output"=w844:i32)  [unwired: 5 in, 1 out]
                  n333 = Divide(x=w844, y=w832) -> (x/y=w821:dbl)
                  n334 = Divide(x=w831, y=w832) -> ()  [unwired: 1 out]
                  n335 = Build Array (concatenate)(w840, w821) -> (w838:dbl[])
                  n336 = Build Array (concatenate)(w845, w821) -> (w843:dbl[])
                  n337 = Build Array (concatenate)(w839, w821) -> (w837:dbl[])
                  n338 = call <instrlib>:"Measure Current.vi"("VISA resource name"=w829, "error in (no error)"=w841) -> ("Measurement"=w827:dbl, "error out"=w830:errorcluster)  [unwired: 11 in, 1 out]
                  n339 = Negate(x=w827) -> (-x=w822:dbl)
                  n340 = Build Array (concatenate)(w826, w822) -> (w825:dbl[])
                  n341 = Bundle(w825, w843) -> (w836:cluster{dbl[], dbl[]})  [unwired: 1 in]
                  n342 = Bundle(w825, w838) -> (w835:cluster{dbl[], dbl[]})  [unwired: 1 in]
                  n343 = Bundle(w825, w837) -> (w834:cluster{dbl[], dbl[]})  [unwired: 1 in]
                  n344 = Build Array(w836, w835, w834) -> (→"Output vs Light":cluster{dbl[], dbl[]}[])
                }
                n345 = call <instrlib>:"ULx Write (Analog 1D DBL 1Chan 1Samp).vi"("task in"=w795, "data"=0.0, "error in"=w797) -> ("task out"=w796:refnum<k24>, "error out"=w798:errorcluster)  [unwired: 10 in, 1 out]
                n346 = call <instrlib>:"ULx Clear Task.vi"("task in"=w796, "error in"=w798) -> ("error out"=w791:errorcluster)  [unwired: 13 in]
              }
            }
          }
          event "Exit": Value Change {
            # "This ensures state is only output if \"OK\" is TRUE. It's not really needed here, since OK has a Latching mechanical action and will reset to FALSE after being read. This merely serves only as an example to show users how one can use Conditional State String."
            # "Exit Button Value Change (pressed) Event\n(this executes Macro: Exit to terminate the VI)"
            n347 = event-data() -> ()  [unwired: 1 in, 1 out]
            n348 = call <vilib>:"Conditional State String__jki_lib_state_machine.vi"("Do State(s)?"="Exit", "State"="Macro: Exit") -> ("State Out"=w850:string)  [unwired: 7 in]
            n349 = call <vilib>:"Add State(s) to Queue__jki_lib_state_machine.vi"("State(s) in Front (\"\")"=w850, "State(s) in (\"\")"=w856) -> ("States Out"=w855:string)  [unwired: 13 in]
          }
          event Panel Close? {
            # "Discard the event because we'll close the front panel ourselves in Macro: Exit"
            # "Close Panel button (pressed) Event\n(this executes Macro: Exit to terminate the VI)"
            n350 = event-data() -> ()  [unwired: 1 in, 1 out]
            n351 = call <vilib>:"Add State(s) to Queue__jki_lib_state_machine.vi"("State(s) in Front (\"\")"="Macro: Exit", "State(s) in (\"\")"=w862) -> ("States Out"=w861:string)  [unwired: 13 in]
            n352 = event-data("Discard?"=TRUE) -> ()  [unwired: 1 in, 1 out]
          }
        }
      }
      frame "---------- Core ----------" {
        # "Do not put any code in this frame.\n(it is a separator no-op)"
        n353 = call <vilib>:"Add State(s) to Queue__jki_lib_state_machine.vi"("State(s) in (\"\")"=w866) -> ("States Out"=w865:string)  [unwired: 14 in]
      }
      frame Default {
        w876 = 42 items=["No error", "Argument error", "Memory is full", "Out of zone", "End of file", "File already open", "Generic file I/O error", "File not found", "File permission error", "Disk is full", "Duplicate path", "Too many files open", "System feature not enabled", "Resource file not found", "Cannot add resource", "Resource not found", "Image not found", "Image memory error", "Pen does not exist", "Config type invalid", "Config token not found", "Config parse error", "Config memory error", "Bad external code format", "Bad external code offset", "External code not present", "Null window", "Destroy window error", "Null menu", "Print aborted", "Bad print record", "Print driver error", "Windows error during printing", "Memory error during printing", "Print dialog error", "Generic print error", "Invalid device refnum", "Device not found", "Device parameter error", "Device unit error", "Cannot open device", "Device call aborted", "Generic error", "Cancelled by user", "Object ID too low", "Object ID too high", "Object not in heap", "Unknown heap", "Unknown object (invalid DefProc)", "Unknown object (DefProc not in table)", "Message out of range", "Invalid (null) method", "Unknown message", "Manager call not supported", "Bad address", "Network operation in progress", "Network operation timed out", "Connection is busy", "Network attribute not supported", "Network error", "Address in use", "System out of memory", "Connection aborted", "Connection refused", "Not connected", "Already connected", "Connection closed", "Initialization error (interapplication manager)", "Bad occurrence", "Wait on unbound occurrence handler", "Occurrence queue overflow", "Datalog type conflict", "Unused", "Unrecognized type (interapplication manager)", "Memory corrupt", "Failed to make temporary DLL", "Old CIN version", "Drag socket not found", "Failed to load drop-object", "Failed to register OLE object", "Failed to release OLE object", "Format specifier type mismatch", "Unknown format specifier", "Too few format specifiers", "Too many format specifiers", "Scan failed", "Newer CIN version", "Error converting to variant", "Runtime menu error", "Password tampered", "Variant attribute not found", "Incompatible variant data type", "Event data is not available", "Event Store is not present", "Occurrence is not found", "Event Queue is not created", "Event info is not available", "Refnum passed is NULL", "Error retrieving Class GUID", "Error retrieving CoClass GUID", "Error retrieving TypeLib GUID.", "Bad built application magic bytes.", "Specific driver is different from the specific driver associated with the Logical Name.", "There is no session opened to the class driver.", "Max Error", "MAX - Error with config objects", "MAX - Error loading configuration", "MAX - Group not supported"]
        # "Current State"
        # "Do not delete, rename, or modify this frame.\n(this is used to capture unhandled states and typos)"
        # "Handle mistyped state name (developer tool)"
        n354 = Format Into String(format string="Software Exception: Unhandled State \"%s\"." ("message"), error in=w872, w867) -> (resulting string=w875:string, error out=w874:errorcluster)  [unwired: 1 in]
        n355 = call <vilib>:"Error Cluster From Error Code.vi"("show call chain? (False)"=TRUE, "error in (no error)"=w874, "error message (\"\")"=w875, "error code (0)"=w876) -> ("error out"=w873:errorcluster)  [unwired: 5 in]
        n356 = call <vilib>:"Add State(s) to Queue__jki_lib_state_machine.vi"("State(s) in (\"\")"=w871) -> ("States Out"=w870:string)  [unwired: 14 in]
      }
      frame "Initialize Core Data" {
        # "Do not delete, rename, or modify this frame.\n(this is used to determine panel behavior on exit)"
        # "originally closed?"
        # "exe?"
        # "If panel starts closed or is an EXE, then close it when we exit"
        n357 = property class="VI"() -> ("FP.State"=w880:T4)  [unwired: 2 in, 2 out]
        n358 = property class="App"() -> ("App.Kind"=w886:T5)  [unwired: 2 in, 2 out]
        n359 = control-ref of="Current VI Reference"() -> (w881:refnum<vi>)
        n360 = Equal?(x=w880, y=T4."Closed" ("Front Panel Window:State")) -> (x = y?=w878:bool)
        n361 = Equal?(x=w886, y=T5."Run Time System" ("Application:Kind")) -> (x = y?=w884:bool)
        n362 = Or(x=w878, y=w884) -> (x .or. y?=w882:bool)
        n363 = Bundle By Name(cluster=w883, "Core.Current VI Reference"=w881, "Core.Close Panel on Exit?"=w882) -> (w888:T8)
        n364 = call <vilib>:"Add State(s) to Queue__jki_lib_state_machine.vi"("State(s) in (\"\")"=w890) -> ("States Out"=w889:string)  [unwired: 14 in]
      }
      frame "Error Handler" {
        # "When running as sourcecode, this function will add previous state data to the error message to aid the developer in troubleshoot errors.\nIf run as an executable, no additional information is added to the error message."
        # "This state receives both Errors and Warnings which is how the Status of this wire can be FALSE"
        # "Unhandled Error -- Display it"
        # "Handle any errors or warnings here.\nYou can also output any states to clean-up after errors or warnings occur"
        # "Clear error or warning"
        n365 = disable-structure shown="Default" {
          disable-tunnel: w896 -> [w903 w904]
          disable-tunnel: w895 -> [w902 _]
          disable-tunnel: [w901 w904] -> w894
          frame condition #0 (active) {
            n366 = call <vilib>:"Append Error Details__jki_lib_state_machine.vi"("error in (no error)"=w903, "Previous State and Argument(s)"=w902) -> ("error out"=w901:errorcluster)  [unwired: 9 in]
          }
          frame condition #1 {
          }
        }
        n367 = call <vilib>:"General Error Handler.vi"("error in (no error)"=w894) -> ()  [unwired: 10 in, 5 out]
        n368 = call-poly <vilib>:"Select State(s)__jki_lib_state_machine.vi"("State(s) if True (\"\")"="/* Post Error States", "Select"=w894, "State(s) if False (\"\")"="/* Post Warning States") -> ("States Out"=w892:string)  [unwired: 12 in]
        n369 = call <vilib>:"Add State(s) to Queue__jki_lib_state_machine.vi"("State(s) in Front (\"\")"=w892, "State(s) in (\"\")"=w900) -> ("States Out"=w899:string)  [unwired: 13 in]
      }
      frame "Exit" {
        # "Do not put any code in this frame.\n(No errors that occur here will be handled.)"
        n370 = call <vilib>:"Add State(s) to Queue__jki_lib_state_machine.vi"("State(s) in (\"\")"=w909) -> ("States Out"=w908:string)  [unwired: 14 in]
      }
      frame "---------- Data ----------" {
        # "Do not put any code in this frame.\n(It is a separator no-op. You can make a copy of this frame to create a new Data frame)"
        n371 = call <vilib>:"Add State(s) to Queue__jki_lib_state_machine.vi"("State(s) in (\"\")"=w913) -> ("States Out"=w912:string)  [unwired: 14 in]
      }
      frame "Data: Initialize" {
        w916 = cluster{"Ramp Pattern":dbl[], dbl[]}[] []  # OpVsCurrent
        w917 = FALSE  # USB3104 connected
        w918 = refnum<k24> refnum  # MWIR CurrentSource
        w919 = refnum<k24> refnum  # SWIR CurrentSource
        w920 = FALSE  # B2901 connected
        w922 = FALSE  # Picoammeter connected
        w923 = refnum<visa-resource-name> "B2901BL"  # B2901 Resource
        w921 = FALSE  # EGSE connected
        w924 = refnum<visa-resource-name> "Picoammeter"  # PicoAmmeter Resource
        w925 = refnum<visa-resource-name> "COM4"  # Detector Resource
        w926 = T11 {"Current VI Reference"=refnum, "Close Panel on Exit?"=FALSE}  # Core
        # "do not delete - used by framework"
        # "Expand Bundle to add new data elements to shift register data."
        # "Data names and types of shift register data are defined by this bundle."
        # "Initialize the shift-register data, here.\n(data names are defined by what you wire into the bundle function)"
        n372 = Bundle("Core"=w926, "Detector Resource"=w925, "EGSE connected"=w921, "PicoAmmeter Resource"=w924, "Picoammeter connected"=w922, "B2901 Resource"=w923, "B2901 connected"=w920, "SWIR CurrentSource"=w919, "MWIR CurrentSource"=w918, "USB3104 connected"=w917, "OpVsCurrent"=w916, "Vout3_Res"="Vout3_Res", "Vout5_Res"="Vout5_Res") -> (w928:T8)  [unwired: 1 in]
        n373 = call <vilib>:"Add State(s) to Queue__jki_lib_state_machine.vi"("State(s) in (\"\")"=w930) -> ("States Out"=w929:string)  [unwired: 14 in]
      }
      frame "Data: Cleanup" {
        # "Cleanup any data and references, here.\n(this is called automatically, by the Macro: Exit)"
        n374 = Unbundle By Name(w931) -> ("Core.Current VI Reference"=w934:refnum<vi>)
        n375 = Close Reference(reference=w934, error in (no error)=w933) -> (error out=w932:errorcluster)
        n376 = call <vilib>:"Add State(s) to Queue__jki_lib_state_machine.vi"("State(s) in (\"\")"=w936) -> ("States Out"=w935:string)  [unwired: 14 in]
      }
      frame "---------- UI ----------" {
        # "Do not put any code in this frame.\n(It is a separator no-op. You can make a copy of this frame to create a new UI frame)"
        n377 = call <vilib>:"Add State(s) to Queue__jki_lib_state_machine.vi"("State(s) in (\"\")"=w940) -> ("States Out"=w939:string)  [unwired: 14 in]
      }
      frame "UI: Initialize" {
        w942 = T6."Disabled and Grayed Out" ("Disabled")
        w944 = FALSE ("connected")
        # "Initialize the User Interface, here.\n(this is called automatically, by the Macro: Initialize)"
        n378 = local read "DecadeSweep"() -> (w941:bool)
        n379 = case shown="False" w941 {
          frame True {
            w951 = T6."Enabled" ("Disabled")
            w952 = T6."Disabled and Grayed Out" ("Disabled")
            n380 = property on="MaxCurrent" class="DigNum (strict)"("DisabledEnum"=w952) -> ()  [unwired: 2 in, 2 out]
            n381 = property on="NPoints" class="DigNum (strict)"("DisabledEnum"=w952) -> ()  [unwired: 2 in, 2 out]
            n382 = property on="NPointsPerDecade" class="Ring (strict)"("DisabledEnum"=w951) -> ()  [unwired: 2 in, 2 out]
            n383 = property on="NumberDecades" class="DigNum (strict)"("DisabledEnum"=w951) -> ()  [unwired: 2 in, 2 out]
          }
          frame False {
            w953 = T6."Disabled and Grayed Out" ("Disabled")
            w954 = T6."Enabled" ("Disabled")
            n384 = property on="MaxCurrent" class="DigNum (strict)"("DisabledEnum"=w954) -> ()  [unwired: 2 in, 2 out]
            n385 = property on="NPoints" class="DigNum (strict)"("DisabledEnum"=w954) -> ()  [unwired: 2 in, 2 out]
            n386 = property on="NPointsPerDecade" class="Ring (strict)"("DisabledEnum"=w953) -> ()  [unwired: 2 in, 2 out]
            n387 = property on="NumberDecades" class="DigNum (strict)"("DisabledEnum"=w953) -> ()  [unwired: 2 in, 2 out]
          }
        }
        n388 = property on="Detector EGSE ID String" class="Str"("Value"="") -> ()  [unwired: 2 in, 2 out]
        n389 = property on="Board Power" class="Bool (strict)"("DisabledEnum"=w942) -> ()  [unwired: 2 in, 2 out]
        n390 = property on="SWIR sweep USB3104" class="Bool"("DisabledEnum"=w942) -> ()  [unwired: 2 in, 2 out]
        n391 = property on="MWIR sweep USB3104" class="Bool"("DisabledEnum"=w942) -> ()  [unwired: 2 in, 2 out]
        n392 = property on="Heater Power" class="Bool (strict)"("DisabledEnum"=w942) -> ()  [unwired: 2 in, 2 out]
        n393 = property on="B2901 Sweep" class="Bool"("DisabledEnum"=w942) -> ()  [unwired: 2 in, 2 out]
        n394 = local write "Heater Power"(w944) -> ()
        n395 = local write "Board Power"(w944) -> ()
        n396 = local write "Pause"(FALSE ("Pause")) -> ()
        n397 = property on="Counts" class="WFChart (strict)"("History Data"=dbl[] []) -> ()  [unwired: 2 in, 2 out]
        n398 = call <vilib>:"Add State(s) to Queue__jki_lib_state_machine.vi"("State(s) in (\"\")"=w950) -> ("States Out"=w949:string)  [unwired: 14 in]
      }
      frame "UI: Uninitialize" {
        # "Cleanup the User Interface, here.\n(this is called automatically, by the Macro: Exit)"
        n399 = call <vilib>:"Add State(s) to Queue__jki_lib_state_machine.vi"("State(s) in (\"\")"=w958) -> ("States Out"=w957:string)  [unwired: 14 in]
      }
      frame "UI: Cursor Set" {
        # "Argument"
        # "Set and Unset Cursor Busy.\n(Usage: \"UI: Cursor Set >> Busy|Idle\")"
        n400 = case shown="\"Idle\", Default" w959 {
          tunnel: w961 -> [w966 w968]
          tunnel: [w965 w967] -> w960
          frame "Idle", Default {
            n401 = call <vilib>:"Unset Busy.vi"("error in (no error)"=w966) -> ("error out"=w965:errorcluster)  [unwired: 10 in]
          }
          frame "Busy" {
            n402 = call <vilib>:"Set Busy.vi"("error in (no error)"=w968) -> ("error out"=w967:errorcluster)  [unwired: 9 in, 1 out]
          }
        }
        n403 = call <vilib>:"Add State(s) to Queue__jki_lib_state_machine.vi"("State(s) in (\"\")"=w964) -> ("States Out"=w963:string)  [unwired: 14 in]
      }
      frame "UI: Front Panel State" {
        # "Argument"
        # "Set Front Panel Open or Closed\n(Usage: \"UI: Front Panel State >> Open|Close\")"
        n404 = Unbundle By Name(w971) -> ("Core.Current VI Reference"=w970:refnum<vi>)
        n405 = case shown="\"Minimize\", \"Minimized\"" w969 {
          tunnel: w973 -> [w981 w996 w1007 w1020 w1033]
          tunnel: [w983 w997 w1009 w1022 w1035] -> w972
          tunnel: w970 -> [w982 w994 w1008 w1021 w1034]
          frame "Open", "Standard", Default {
            w976 = T4."Standard" ("State")
            n406 = property class="VI"(reference=w982, error in=w981) -> (reference out=w979:refnum<vi>, error out=w980:errorcluster, "FP.State"=w978:T4)
            n407 = Not Equal?(x=w978, y=w976) -> (x != y?=w977:bool)
            n408 = case shown="True" w977 {
              tunnel: [w987 w989] -> w983
              tunnel: w980 -> [w986 w989]
              tunnel: w979 -> [w985 _]
              tunnel: w976 -> [w984 _]
              frame True {
                n409 = invoke class="VI" method="FP.Open"(reference=w985, error in=w986, "Activate"=TRUE, "State"=w984) -> (error out=w987:errorcluster)  [unwired: 1 in, 4 out]
              }
              frame False {
              }
            }
          }
          frame "Close", "Closed" {
            n410 = property class="VI"(reference=w994, error in=w996) -> (reference out=w993:refnum<vi>, error out=w995:errorcluster, "FP.State"=w991:T4)
            n411 = Not Equal?(x=w991, y=T4."Closed" ("Front Panel Window:State")) -> (x != y?=w990:bool)
            n412 = case shown="True" w990 {
              tunnel: [w998 w1001] -> w997
              tunnel: w995 -> [w998 w1000]
              tunnel: w993 -> [_ w999]
              frame False {
              }
              frame True {
                n413 = invoke class="VI" method="FP.Close"(reference=w999, error in=w1000) -> (error out=w1001:errorcluster)  [unwired: 1 in, 2 out]
              }
            }
          }
          frame "Hidden", "Hide" {
            w1002 = T4."Hidden" ("State")
            n414 = property class="VI"(reference=w1008, error in=w1007) -> (reference out=w1005:refnum<vi>, error out=w1006:errorcluster, "FP.State"=w1004:T4)
            n415 = Not Equal?(x=w1004, y=w1002) -> (x != y?=w1003:bool)
            n416 = case shown="True" w1003 {
              tunnel: [w1013 w1014] -> w1009
              tunnel: w1006 -> [w1012 w1014]
              tunnel: w1005 -> [w1011 _]
              tunnel: w1002 -> [w1010 _]
              frame True {
                n417 = invoke class="VI" method="FP.Open"(reference=w1011, error in=w1012, "State"=w1010) -> (error out=w1013:errorcluster)  [unwired: 2 in, 4 out]
              }
              frame False {
              }
            }
          }
          frame "Minimize", "Minimized" {
            w1015 = T4."Minimized" ("State")
            n418 = property class="VI"(reference=w1021, error in=w1020) -> (reference out=w1018:refnum<vi>, error out=w1019:errorcluster, "FP.State"=w1017:T4)
            n419 = Not Equal?(x=w1017, y=w1015) -> (x != y?=w1016:bool)
            n420 = case shown="True" w1016 {
              tunnel: [w1026 w1027] -> w1022
              tunnel: w1019 -> [w1025 w1027]
              tunnel: w1018 -> [w1024 _]
              tunnel: w1015 -> [w1023 _]
              frame True {
                n421 = invoke class="VI" method="FP.Open"(reference=w1024, error in=w1025, "State"=w1023) -> (error out=w1026:errorcluster)  [unwired: 2 in, 4 out]
              }
              frame False {
              }
            }
          }
          frame "Maximize", "Maximized" {
            w1028 = T4."Maximized" ("State")
            n422 = property class="VI"(reference=w1034, error in=w1033) -> (reference out=w1031:refnum<vi>, error out=w1032:errorcluster, "FP.State"=w1030:T4)
            n423 = Not Equal?(x=w1030, y=w1028) -> (x != y?=w1029:bool)
            n424 = case shown="True" w1029 {
              tunnel: [w1039 w1040] -> w1035
              tunnel: w1032 -> [w1038 w1040]
              tunnel: w1031 -> [w1037 _]
              tunnel: w1028 -> [w1036 _]
              frame True {
                n425 = invoke class="VI" method="FP.Open"(reference=w1037, error in=w1038, "State"=w1036) -> (error out=w1039:errorcluster)  [unwired: 2 in, 4 out]
              }
              frame False {
              }
            }
          }
        }
        n426 = call <vilib>:"Add State(s) to Queue__jki_lib_state_machine.vi"("State(s) in (\"\")"=w975) -> ("States Out"=w974:string)  [unwired: 14 in]
      }
      frame "---------- Macro ----------" {
        # "Do not put any code in this frame.\n(It is a separator no-op. You can make a copy of this frame to create a new Macro frame)"
        n427 = call <vilib>:"Add State(s) to Queue__jki_lib_state_machine.vi"("State(s) in (\"\")"=w1044) -> ("States Out"=w1043:string)  [unwired: 14 in]
      }
      frame "Macro: Initialize" {
        w1045 = "Data: Initialize\nInitialize Core Data\nUI: Initialize\nUI: Front Panel State >> Open"  # Data: Initialize Initialize Core Data UI: Initialize UI: Front Panel State >> Open
        # "Initialization Macro\n(This is called once, when the VI starts)"
        n428 = call <vilib>:"Add State(s) to Queue__jki_lib_state_machine.vi"("State(s) in Front (\"\")"=w1045, "State(s) in (\"\")"=w1049) -> ("States Out"=w1048:string)  [unwired: 13 in]
      }
      frame "Macro: Exit" {
        # "Exit Macro\n(This is called once, when the VI exits)"
        n429 = Unbundle By Name(w1056) -> ("Core.Close Panel on Exit?"=w1051:bool)
        n430 = call <vilib>:"Conditional State String__jki_lib_state_machine.vi"("Do State(s)?"=w1051, "State"="UI: Front Panel State >> Close") -> ("State Out"=w1050:string)  [unwired: 7 in]
        n431 = call <vilib>:"Add State(s) to Queue__jki_lib_state_machine.vi"("State(s) in (\"\")"=w1050, "State(s) at Back (\"\")"="UI: Uninitialize\nData: Cleanup\nHardware: Close EGSE\nHardware: Close PicoAmmeter\nHardware: Close B2901\nHardware: Close USB3104\nExit") -> ("States Out"=w1054:string)  [unwired: 13 in]
        n432 = call <vilib>:"Add State(s) to Queue__jki_lib_state_machine.vi"("State(s) in Front (\"\")"=w1054, "State(s) in (\"\")"=w1058) -> ("States Out"=w1057:string)  [unwired: 13 in]
      }
      frame "---------- Hardware ----------" {
        # "Template Separator\n(You can make a copy of, or modify, this frame)"
        n433 = call <vilib>:"Add State(s) to Queue__jki_lib_state_machine.vi"("State(s) in (\"\")"=w1062) -> ("States Out"=w1061:string)  [unwired: 14 in]
      }
      frame "Hardware: Init PicoAmmeter" {
        n434 = call "Keithley 648X Series SetupAcquisition.vi"("error in (no error)"=w1068, "VISA resource name"="PicoAmmeter VISA") -> ("error out"=w1067:errorcluster, "VISA resource name out"=w1064:refnum<visa-resource-name>)  [unwired: 7 in]
        n435 = case shown="No Error" w1067 {
          selector: w1067 -> [w1074 w1080]
          tunnel: w1066 -> [w1077 w1081]
          tunnel: [w1076 w1081] -> w1065
          tunnel: w1064 -> [w1075 _]
          tunnel: [w1074 w1078] -> w1063
          frame No Error {
            n436 = Bundle By Name(cluster=w1077, "Picoammeter connected"=TRUE, "PicoAmmeter Resource"=w1075) -> (w1076:T8)
            "PicoAmmeter Connected" <- TRUE ("PicoAmmeter Connected")
          }
          frame Error {
            n437 = One Button Dialog(message="Can't find Picoammeter\nPlease Check connections and VISA name\nbefore trying again") -> ()  [unwired: 1 in, 1 out]
            n438 = call <vilib>:"Clear Errors.vi"("error in (no error)"=w1080) -> ("error out"=w1078:errorcluster)  [unwired: 5 in, 1 out]
          }
        }
        n439 = call <vilib>:"Add State(s) to Queue__jki_lib_state_machine.vi"("State(s) in (\"\")"=w1071) -> ("States Out"=w1070:string)  [unwired: 14 in]
      }
      frame "Hardware: Init B2901" {
        n440 = call <instrlib>:"Initialize.vi"("error in (no error)"=w1084, "ID Query (True)"=FALSE, "VISA resource name"="B2901BL VISA") -> ("error out"=w1085:errorcluster, "VISA resource name out"=w1083:refnum<visa-resource-name>)  [unwired: 7 in]
        n441 = case shown="No Error" w1085 {
          selector: w1085 -> [w1097 w1116]
          tunnel: w1089 -> [w1113 w1117]
          tunnel: [w1112 w1117] -> w1086
          tunnel: w1083 -> [w1096 _]
          tunnel: [w1092 w1114] -> w1082
          frame No Error {
            w1102 = u16 50 items=["60 Hz"=60, "50 Hz or 400 Hz"=50] ("Power Line Frequency  (60 Hz)")
            w1100 = u16 1 items=["Volts", "Current", "Resistance"] ("Function (0: Volts)")
            w1098 = u16 0 items=["Volts", "Current", "Resistance"] ("Function (0: Volts)")
            # "Set defaults on B2901BL"
            n442 = call <instrlib>:"Configure Power Line Frequency.vi"("error in (no error)"=w1097, "Power Line Frequency  (60 Hz)"=w1102, "VISA resource name"=w1096) -> ("error out"=w1106:errorcluster, "VISA resource name out"=w1107:refnum<visa-resource-name>)  [unwired: 7 in]
            n443 = call <instrlib>:"Configure Measurement.vi"("error in (no error)"=w1106, "Enable Auto Range (T:Enable)"=TRUE, "Function (0: Volts)"=w1098, "VISA resource name"=w1107) -> ("error out"=w1108:errorcluster, "VISA resource name out"=w1109:refnum<visa-resource-name>)  [unwired: 6 in]
            n444 = call <instrlib>:"Configure Measurement.vi"("error in (no error)"=w1108, "Enable Auto Range (T:Enable)"=TRUE, "Function (0: Volts)"=w1100, "VISA resource name"=w1109) -> ("error out"=w1105:errorcluster, "VISA resource name out"=w1104:refnum<visa-resource-name>)  [unwired: 6 in]
            n445 = VISA Write(VISA resource name=w1104, write buffer=":SOUR:CURR:RANGE 1e-4", error in (no error)=w1105) -> (VISA resource name out=w1095:refnum<visa-resource-name>, error out=w1093:errorcluster)  [unwired: 1 out]
            n446 = property on="B2901 Sweep" class="Bool"(error in=w1093, "DisabledEnum"=T6."Enabled" ("Disabled")) -> (error out=w1092:errorcluster)  [unwired: 1 in, 1 out]
            n447 = Bundle By Name(cluster=w1113, "B2901 connected"=TRUE ("ISource connected"), "B2901 Resource"=w1095) -> (w1112:T8)
            "B2901BL Connected" <- TRUE ("ISource Connected")
          }
          frame Error {
            n448 = One Button Dialog(message="Can't find B2901BL\nPlease Check connections and VISA name\nbefore trying again") -> ()  [unwired: 1 in, 1 out]
            n449 = call <vilib>:"Clear Errors.vi"("error in (no error)"=w1116) -> ("error out"=w1114:errorcluster)  [unwired: 5 in, 1 out]
          }
        }
        n450 = call <vilib>:"Add State(s) to Queue__jki_lib_state_machine.vi"("State(s) in (\"\")"=w1091) -> ("States Out"=w1090:string)  [unwired: 14 in]
      }
      frame "Hardware: Init USB3104" {
        n451 = call-poly <instrlib>:"ULx Create Virtual Channel.vi"("maximum value"=10.0, "minimum value"=0.0, "physical channels"="USB3104 VOut3 (SWIR)", "error in"=w1134) -> ("task out"=w1125:refnum<k24>, "error out"=w1127:errorcluster)  [unwired: 10 in]
        n452 = call <instrlib>:"ULx Write (Analog 1D DBL 1Chan 1Samp).vi"("task in"=w1125, "data"=0.0, "error in"=w1127) -> ("task out"=w1123:refnum<k24>, "error out"=w1126:errorcluster)  [unwired: 10 in, 1 out]
        n453 = call-poly <instrlib>:"ULx Create Virtual Channel.vi"("maximum value"=10.0, "minimum value"=0.0, "physical channels"="USB3104 VOut5 (MWIR)", "error in"=w1126) -> ("task out"=w1119:refnum<k24>, "error out"=w1121:errorcluster)  [unwired: 10 in]
        n454 = call <instrlib>:"ULx Write (Analog 1D DBL 1Chan 1Samp).vi"("task in"=w1119, "data"=0.0, "error in"=w1121) -> ("task out"=w1120:refnum<k24>, "error out"=w1122:errorcluster)  [unwired: 10 in, 1 out]
        n455 = case shown="No Error" w1122 {
          selector: w1122 -> [w1143 w1150]
          tunnel: w1137 -> [w1147 w1151]
          tunnel: [w1146 w1151] -> w1136
          tunnel: w1123 -> [w1142 _]
          tunnel: [w1143 w1148] -> w1135
          tunnel: w1120 -> [w1141 _]
          frame No Error {
            w1140 = T6."Enabled" ("Disabled")
            n456 = property on="SWIR sweep USB3104" class="Bool"("DisabledEnum"=w1140) -> ()  [unwired: 2 in, 2 out]
            n457 = property on="MWIR sweep USB3104" class="Bool"("DisabledEnum"=w1140) -> ()  [unwired: 2 in, 2 out]
            n458 = property on="Vout3 Sweep" class="Bool"("DisabledEnum"=w1140) -> ()  [unwired: 2 in, 2 out]
            n459 = property on="Vout5 sweep" class="Bool"("DisabledEnum"=w1140) -> ()  [unwired: 2 in, 2 out]
            n460 = Bundle By Name(cluster=w1147, "SWIR CurrentSource"=w1142, "USB3104 connected"=TRUE ("ISource connected"), "MWIR CurrentSource"=w1141) -> (w1146:T8)
            "USB3104 Connected" <- TRUE ("ISource Connected")
          }
          frame Error {
            n461 = One Button Dialog(message="Can't find USB-3104\nPlease Check connections and Device dropdowns\nbefore trying again\nYou may need to run Instalcal after USB3104 Installation") -> ()  [unwired: 1 in, 1 out]
            n462 = call <vilib>:"Clear Errors.vi"("error in (no error)"=w1150) -> ("error out"=w1148:errorcluster)  [unwired: 5 in, 1 out]
          }
        }
        n463 = call <vilib>:"Add State(s) to Queue__jki_lib_state_machine.vi"("State(s) in (\"\")"=w1139) -> ("States Out"=w1138:string)  [unwired: 14 in]
      }
      frame "Hardware: Init EGSE" {
        n464 = call <instrlib>:"Initialize.vi"("Serial Configuration"=T7 {"Baud Rate"=57600, "Parity"=0, "Data Bits"=8, "Stop Bits"=10, "Flow Control"=0}, "error in (no error)"=w1155, "VISA resource name"="Detector VISA") -> ("error out"=w1154:errorcluster, "ID String"=→"Detector EGSE ID String":string, "VISA resource name out"=w1160:refnum<visa-resource-name>)  [unwired: 6 in]
        n465 = case shown="No Error" w1154 {
          selector: w1154 -> [w1173 w1186]
          tunnel: w1160 -> [w1178 _]
          tunnel: [w1171 w1187] -> w1156
          tunnel: w1153 -> [w1177 w1189]
          tunnel: [w1176 w1189] -> w1152
          frame No Error {
            w1170 = T6."Enabled" ("Disabled")
            n466 = local read "Oversample"() -> (w1179:i32)
            n467 = local read "SPI Clock"() -> (w1184:i64)
            n468 = call <instrlib>:"Set OverSample.vi"("error in (no error)"=w1173, "oversample (0)"=w1179, "VISA resource name"=w1178) -> ("error out"=w1180:errorcluster, "VISA resource name out"=w1182:refnum<visa-resource-name>)  [unwired: 7 in]
            n469 = call <instrlib>:"Set Clock.vi"("error in (no error)"=w1180, "ClockSpeed"=w1184, "VISA resource name"=w1182) -> ("error out"=w1181:errorcluster, "VISA resource name out"=w1183:refnum<visa-resource-name>)  [unwired: 7 in]
            n470 = local read "SWIR DAC"() -> (w1185:i32)
            n471 = call <instrlib>:"Set DAC.vi"("error in (no error)"=w1181, "value (0)"=w1185, "chan (0)"=0, "VISA resource name"=w1183) -> ("error out"=w1169:errorcluster, "VISA resource name out"=w1166:refnum<visa-resource-name>)  [unwired: 6 in]
            n472 = local read "MWIR DAC"() -> (w1164:i32)
            n473 = call <instrlib>:"Set DAC.vi"("error in (no error)"=w1169, "value (0)"=w1164, "chan (0)"=1, "VISA resource name"=w1166) -> ("error out"=w1168:errorcluster, "VISA resource name out"=w1163:refnum<visa-resource-name>)  [unwired: 6 in]
            n474 = Bundle By Name(cluster=w1177, "EGSE connected"=TRUE, "Detector Resource"=w1163) -> (w1176:T8)
            n475 = property on="Board Power" class="Bool (strict)"(error in=w1168, "DisabledEnum"=w1170) -> (error out=w1172:errorcluster)  [unwired: 1 in, 1 out]
            n476 = property on="Heater Power" class="Bool (strict)"(error in=w1172, "DisabledEnum"=w1170) -> (error out=w1171:errorcluster)  [unwired: 1 in, 1 out]
            "EGSE Connected" <- TRUE ("Connected")
          }
          frame Error {
            n477 = One Button Dialog(message="Can't find EGSE\nPlease Check connections and VISA name\nbefore trying again") -> ()  [unwired: 1 in, 1 out]
            n478 = call <vilib>:"Clear Errors.vi"("error in (no error)"=w1186) -> ("error out"=w1187:errorcluster)  [unwired: 5 in, 1 out]
          }
        }
        n479 = call <vilib>:"Add State(s) to Queue__jki_lib_state_machine.vi"("State(s) in (\"\")"=w1162) -> ("States Out"=w1161:string)  [unwired: 14 in]
      }
      frame "Hardware: Close EGSE" {
        n480 = Unbundle By Name(w1193) -> ("Detector Resource"=w1194:refnum<visa-resource-name>, "EGSE connected"=w1190:bool)
        n481 = case shown="True" w1190 {
          tunnel: w1195 -> [w1198 w1217]
          tunnel: w1194 -> [_ w1216]
          tunnel: w1193 -> [w1199 w1215]
          tunnel: [w1199 w1214] -> w1192
          tunnel: [w1198 w1206] -> w1191
          frame False {
          }
          frame True {
            w1205 = T6."Disabled and Grayed Out" ("Disabled")
            n482 = call <instrlib>:"Set Power.vi"("error in (no error)"=w1217, "Power (0)"=FALSE, "VISA resource name"=w1216) -> ("error out"=w1201:errorcluster, "VISA resource name out"=w1204:refnum<visa-resource-name>)  [unwired: 7 in]
            n483 = call <instrlib>:"Set Heater.vi"("error in (no error)"=w1201, "Power (0)"=FALSE, "VISA resource name"=w1204) -> ("error out"=w1202:errorcluster, "VISA resource name out"=w1203:refnum<visa-resource-name>)  [unwired: 7 in]
            n484 = property on="Board Power" class="Bool (strict)"(error in=w1202, "Value"=FALSE ("Power")) -> (error out=w1220:errorcluster)  [unwired: 1 in, 1 out]
            n485 = call <instrlib>:"Close.vi"("error in (no error)"=w1220, "VISA resource name"=w1203) -> ("error out"=w1211:errorcluster)  [unwired: 9 in]
            n486 = property on="Detector EGSE ID String" class="Str"(error in=w1211, "Value"="") -> (error out=w1210:errorcluster)  [unwired: 1 in, 1 out]
            n487 = property on="EGSE Connected" class="Bool (strict)"(error in=w1210, "Value"=FALSE ("Connected")) -> (error out=w1208:errorcluster)  [unwired: 1 in, 1 out]
            n488 = Bundle By Name(cluster=w1215, "EGSE connected"=FALSE) -> (w1214:T8)
            n489 = property on="Board Power" class="Bool (strict)"(error in=w1208, "DisabledEnum"=w1205) -> (error out=w1207:errorcluster)  [unwired: 1 in, 1 out]
            n490 = property on="Heater Power" class="Bool (strict)"(error in=w1207, "DisabledEnum"=w1205) -> (error out=w1206:errorcluster)  [unwired: 1 in, 1 out]
          }
        }
        n491 = call <vilib>:"Add State(s) to Queue__jki_lib_state_machine.vi"("State(s) in (\"\")"=w1197) -> ("States Out"=w1196:string)  [unwired: 14 in]
      }
      frame "Hardware: Close PicoAmmeter" {
        n492 = Unbundle By Name(w1224) -> ("Picoammeter connected"=w1221:bool, "PicoAmmeter Resource"=w1225:refnum<visa-resource-name>)
        n493 = case shown="True" w1221 {
          tunnel: w1226 -> [w1229 w1232]
          tunnel: w1225 -> [_ w1231]
          tunnel: w1224 -> [w1230 w1238]
          tunnel: [w1230 w1237] -> w1223
          tunnel: [w1229 w1234] -> w1222
          frame False {
          }
          frame True {
            n494 = Bundle By Name(cluster=w1238, "Picoammeter connected"=FALSE ("EGSE connected")) -> (w1237:T8)
            n495 = call <instrlib>:"Close.vi"("error in (no error)"=w1232, "VISA resource name"=w1231) -> ("error out"=w1235:errorcluster)  [unwired: 9 in]
            n496 = property on="PicoAmmeter Connected" class="Bool (strict)"(error in=w1235, "Value"=FALSE ("Connected")) -> (error out=w1234:errorcluster)  [unwired: 1 in, 1 out]
          }
        }
        n497 = call <vilib>:"Add State(s) to Queue__jki_lib_state_machine.vi"("State(s) in (\"\")"=w1228) -> ("States Out"=w1227:string)  [unwired: 14 in]
      }
      frame "Hardware: Close B2901" {
        n498 = Unbundle By Name(w1244) -> ("B2901 connected"=w1240:bool, "B2901 Resource"=w1241:refnum<visa-resource-name>)
        n499 = case shown="True" w1240 {
          tunnel: w1244 -> [w1247 w1265]
          tunnel: [w1247 w1264] -> w1239
          tunnel: [w1248 w1262] -> w1243
          tunnel: w1242 -> [w1248 w1255]
          tunnel: w1241 -> [_ w1254]
          frame False {
          }
          frame True {
            w1257 = u16 1 items=["Voltage", "Current"] ("Source Mode  (0: Voltage)")
            n500 = call <instrlib>:"Configure Output.vi"("Source Mode  (0: Voltage)"=w1257, "error in (no error)"=w1255, "Output Level (0)"=0.0, "VISA resource name"=w1254) -> ("error out"=w1259:errorcluster, "VISA resource name out"=w1260:refnum<visa-resource-name>)  [unwired: 6 in]
            n501 = call <instrlib>:"Enable Output.vi"("error in (no error)"=w1259, "Enable Output (T: Enable)"=TRUE ("Auto Output-Off (F: Disable)"), "VISA resource name"=w1260) -> ("error out"=w1252:errorcluster, "VISA resource name out"=w1253:refnum<visa-resource-name>)  [unwired: 7 in]
            n502 = call <instrlib>:"Close.vi"("error in (no error)"=w1252, "VISA resource name"=w1253) -> ("error out"=w1250:errorcluster)  [unwired: 9 in]
            n503 = property on="B2901 Sweep" class="Bool"(error in=w1250, "DisabledEnum"=T6."Disabled and Grayed Out" ("Disabled")) -> (error out=w1249:errorcluster)  [unwired: 1 in, 1 out]
            n504 = Bundle By Name(cluster=w1265, "B2901 connected"=FALSE ("EGSE connected")) -> (w1264:T8)
            n505 = property on="B2901BL Connected" class="Bool (strict)"(error in=w1249, "Value"=FALSE ("Connected")) -> (error out=w1262:errorcluster)  [unwired: 1 in, 1 out]
          }
        }
        n506 = call <vilib>:"Add State(s) to Queue__jki_lib_state_machine.vi"("State(s) in (\"\")"=w1246) -> ("States Out"=w1245:string)  [unwired: 14 in]
      }
      frame "Hardware: Close USB3104" {
        n507 = Unbundle By Name(w1272) -> ("USB3104 connected"=w1267:bool, "SWIR CurrentSource"=w1268:refnum<k24>, "MWIR CurrentSource"=w1266:refnum<k24>)
        n508 = case shown="True" w1267 {
          tunnel: w1272 -> [w1275 w1291]
          tunnel: [w1275 w1290] -> w1271
          tunnel: [w1276 w1288] -> w1270
          tunnel: w1269 -> [w1276 w1286]
          tunnel: w1268 -> [_ w1283]
          tunnel: w1266 -> [_ w1285]
          frame False {
          }
          frame True {
            w1277 = T6."Disabled and Grayed Out" ("Disabled")
            n509 = call <instrlib>:"ULx Clear Task.vi"("task in"=w1285, "error in"=w1286) -> ("error out"=w1284:errorcluster)  [unwired: 13 in]
            n510 = call <instrlib>:"ULx Clear Task.vi"("task in"=w1283, "error in"=w1284) -> ("error out"=w1282:errorcluster)  [unwired: 13 in]
            n511 = property on="SWIR sweep USB3104" class="Bool"(error in=w1282, "DisabledEnum"=w1277) -> (error out=w1281:errorcluster)  [unwired: 1 in, 1 out]
            n512 = property on="MWIR sweep USB3104" class="Bool"(error in=w1281, "DisabledEnum"=w1277) -> (error out=w1280:errorcluster)  [unwired: 1 in, 1 out]
            n513 = Bundle By Name(cluster=w1291, "USB3104 connected"=FALSE ("EGSE connected")) -> (w1290:T8)
            n514 = property on="Vout3 Sweep" class="Bool"(error in=w1280, "DisabledEnum"=w1277) -> (error out=w1279:errorcluster)  [unwired: 1 in, 1 out]
            n515 = property on="Vout5 Sweep" class="Bool"(error in=w1279, "DisabledEnum"=w1277) -> (error out=w1278:errorcluster)  [unwired: 1 in, 1 out]
            n516 = property on="USB3104 Connected" class="Bool (strict)"(error in=w1278, "Value"=FALSE ("Connected")) -> (error out=w1288:errorcluster)  [unwired: 1 in, 1 out]
          }
        }
        n517 = call <vilib>:"Add State(s) to Queue__jki_lib_state_machine.vi"("State(s) in (\"\")"=w1274) -> ("States Out"=w1273:string)  [unwired: 14 in]
      }
    }
  }
